vi "Periodic Tasks.vi"(8 "error in":errorcluster) -> (0 "error out":errorcluster)   [LabVIEW 2018]
doc: "This VI runs in parallel to other tasks. It can contain as many user-defined periodic loops as you need. These can carry out PID or other sorts of timed response."
uses:
  <vilib>/Rock Robotics/WPI/Joystick/WPI_JoystickDevRef.ctl
  <vilib>/Rock Robotics/WPI/Joystick/WPI_JoystickDeviceEnum.ctl
  <vilib>/Rock Robotics/WPI/RobotDrive/WPI_RobotDriveDevRef.ctl
  <vilib>/Rock Robotics/WPI/MotorControl/WPI_MotorControlDeviceRef.ctl
  <vilib>/Rock Robotics/WPI/MotorControl/WPI_MotorControlType.ctl
  <vilib>/Rock Robotics/SystemInterfaces/DIO/FPGA_DIOPWMChannel.ctl
  <vilib>/Rock Robotics/WPI/PWM/WPI_PWMDeadband.ctl
  <vilib>/Rock Robotics/SystemInterfaces/DIO/FPGA_DIOChannel.ctl
  <vilib>/Rock Robotics/WPI/Solenoid/WPI_SolenoidDevRef.ctl
  <vilib>/Rock Robotics/WPI/Solenoid/WPI_SolenoidChannel.ctl
  <vilib>/Rock Robotics/WPI/DigitalInput/WPI_DigitalInputDevRef.ctl
  Vision States.ctl
  <vilib>/Rock Robotics/WPI/DriverStation/WPI_DriverStationRobotMode2.ctl
  Hatch Retainer States.ctl
  HAB Bk Spd Motor States.ctl
  Hatch Kicking States.ctl
  <vilib>/Rock Robotics/WPI/ThirdParty/Phoenix-LabVIEW/Motor Controller/Controls/CTRE_Phoenix_MotorControl_MotionProfileTrajectoryPoint.ctl
  <vilib>/Rock Robotics/WPI/Utilities/WPI_GetSetVariantRefNum.vi
  <vilib>/Rock Robotics/WPI/ThirdParty/Phoenix-LabVIEW/Motor Controller/Get/CTRE_Phoenix_MotorController_GetQuadratureData.vi
  Robot Global Data.vi
  <vilib>/Rock Robotics/Network Tables/NT Write Number.vi
  <vilib>/Rock Robotics/WPI/ThirdParty/Phoenix-LabVIEW/Motor Controller/Closed Loop/Motion Profile/CTRE_Phoenix_MotorControl_BufferedTrajectoryPointStream_WriteAll.vi
  <vilib>/Rock Robotics/Network Tables/NT Read Number.vi
  <vilib>/Rock Robotics/WPI/Solenoid/WPI_SolenoidValue.ctl
  <vilib>/Rock Robotics/WPI/Solenoid/WPI_SolenoidSetEnum.vi
  <vilib>/addons/control/pid/NI_PID_pid.lvlib
  <vilib>/Rock Robotics/WPI/ThirdParty/Phoenix-LabVIEW/Motor Controller/Controls/CTRE_Phoenix_MotorControl_ControlMode.ctl
  <vilib>/addons/control/pid/pid.llb/PID (DBL).vi
  <vilib>/Rock Robotics/Network Tables/NT Write Boolean.vi
panel:
  in  "HAB3DriveModuleMotorDevRef 2":T1={"DeviceStatus"={"status"=FALSE, "code"=0, "source"=""}, "Type"=enum."PWM", "PWM"={"PWM Channel"=enum."Invalid", "DeadBand"={"Name"="", "maxPositivePwm"=0, "minPositivePwm"=0, "centerPwm"=0, "maxNegativePwm"=0, "minNegativePwm"=0, "angularRange"=0}}, "CAN"={"Device Number"=0, "SetOutput VI Ref"=variant(refnum<vi> refnum), "GetOutput VI Ref"=variant(refnum<vi> refnum), "Enable VI Ref"=variant(refnum<vi> refnum), "Disable VI Ref"=variant(refnum<vi> refnum), "Data"=variant}, "Invert"=FALSE, "DIO PWM"={"PWM \"Enable\" Channel"=enum."Invalid", "DIOChannel"=enum."Invalid", "PWM Rate"=0.0}}
  in  "BkSpdAdjusterMotorDevRef":T1={"DeviceStatus"={"status"=FALSE, "code"=0, "source"=""}, "Type"=enum."PWM", "PWM"={"PWM Channel"=enum."Invalid", "DeadBand"={"Name"="", "maxPositivePwm"=0, "minPositivePwm"=0, "centerPwm"=0, "maxNegativePwm"=0, "minNegativePwm"=0, "angularRange"=0}}, "CAN"={"Device Number"=0, "SetOutput VI Ref"=variant(refnum<vi> refnum), "GetOutput VI Ref"=variant(refnum<vi> refnum), "Enable VI Ref"=variant(refnum<vi> refnum), "Disable VI Ref"=variant(refnum<vi> refnum), "Data"=variant}, "Invert"=FALSE, "DIO PWM"={"PWM \"Enable\" Channel"=enum."Invalid", "DIOChannel"=enum."Invalid", "PWM Rate"=0.0}}
  in  "HABAssisterSolenoidDevRef":T6={"DevStatus"={"status"=FALSE, "code"=0, "source"=""}, "Pneumatics Control Module"=0, "Forward Solenoid Channel"=enum."Invalid", "Reverse Solenoid Channel"=enum."Invalid"}
  out "Right Traj. Pts Array":dbl[][](array[numeric])
  out "Left Traj. Pts Array":dbl[][](array[numeric])
  in  "Back HAB 3 Limit Switch":T8={"DevStatus"={"status"=FALSE, "code"=0, "source"=""}, "DIO Channel"=enum."Invalid"}
  in  "Front HAB 3 Limit Switch":T8={"DevStatus"={"status"=FALSE, "code"=0, "source"=""}, "DIO Channel"=enum."Invalid"}
  in  "BottomRetainerSwitchDevRef":T8={"DevStatus"={"status"=FALSE, "code"=0, "source"=""}, "DIO Channel"=enum."Invalid"}
  in  "TopRetainerSwitchDevRef":T8={"DevStatus"={"status"=FALSE, "code"=0, "source"=""}, "DIO Channel"=enum."Invalid"}
  in  "HatchRetainerMotorDevRef":T1={"DeviceStatus"={"status"=FALSE, "code"=0, "source"=""}, "Type"=enum."PWM", "PWM"={"PWM Channel"=enum."Invalid", "DeadBand"={"Name"="", "maxPositivePwm"=0, "minPositivePwm"=0, "centerPwm"=0, "maxNegativePwm"=0, "minNegativePwm"=0, "angularRange"=0}}, "CAN"={"Device Number"=0, "SetOutput VI Ref"=variant(refnum<vi> refnum), "GetOutput VI Ref"=variant(refnum<vi> refnum), "Enable VI Ref"=variant(refnum<vi> refnum), "Disable VI Ref"=variant(refnum<vi> refnum), "Data"=variant}, "Invert"=FALSE, "DIO PWM"={"PWM \"Enable\" Channel"=enum."Invalid", "DIOChannel"=enum."Invalid", "PWM Rate"=0.0}}
  in  "HAB3BackSolenoidDevRef":T6={"DevStatus"={"status"=FALSE, "code"=0, "source"=""}, "Pneumatics Control Module"=0, "Forward Solenoid Channel"=enum."Invalid", "Reverse Solenoid Channel"=enum."Invalid"}
  in  "HAB3FrontSolenoidDevRef":T6={"DevStatus"={"status"=FALSE, "code"=0, "source"=""}, "Pneumatics Control Module"=0, "Forward Solenoid Channel"=enum."Invalid", "Reverse Solenoid Channel"=enum."Invalid"}
  in  "AuxJoystickDevRef":T9={"Device"=enum."USB 1"}
  in  "DriveJoystickDevRef":T9={"Device"=enum."USB 1"}
  in  "HAB3DriveModuleMotorDevRef":T1={"DeviceStatus"={"status"=FALSE, "code"=0, "source"=""}, "Type"=enum."PWM", "PWM"={"PWM Channel"=enum."Invalid", "DeadBand"={"Name"="", "maxPositivePwm"=0, "minPositivePwm"=0, "centerPwm"=0, "maxNegativePwm"=0, "minNegativePwm"=0, "angularRange"=0}}, "CAN"={"Device Number"=0, "SetOutput VI Ref"=variant(refnum<vi> refnum), "GetOutput VI Ref"=variant(refnum<vi> refnum), "Enable VI Ref"=variant(refnum<vi> refnum), "Disable VI Ref"=variant(refnum<vi> refnum), "Data"=variant}, "Invert"=FALSE, "DIO PWM"={"PWM \"Enable\" Channel"=enum."Invalid", "DIOChannel"=enum."Invalid", "PWM Rate"=0.0}}
  in  "LifterSolenoidDevRef":T6={"DevStatus"={"status"=FALSE, "code"=0, "source"=""}, "Pneumatics Control Module"=0, "Forward Solenoid Channel"=enum."Invalid", "Reverse Solenoid Channel"=enum."Invalid"}
  in  "DriveJoystickDevRef":T9={"Device"=enum."USB 1"}
  in  "HatchCollectorMotorDevRef":T1={"DeviceStatus"={"status"=FALSE, "code"=0, "source"=""}, "Type"=enum."PWM", "PWM"={"PWM Channel"=enum."Invalid", "DeadBand"={"Name"="", "maxPositivePwm"=0, "minPositivePwm"=0, "centerPwm"=0, "maxNegativePwm"=0, "minNegativePwm"=0, "angularRange"=0}}, "CAN"={"Device Number"=0, "SetOutput VI Ref"=variant(refnum<vi> refnum), "GetOutput VI Ref"=variant(refnum<vi> refnum), "Enable VI Ref"=variant(refnum<vi> refnum), "Disable VI Ref"=variant(refnum<vi> refnum), "Data"=variant}, "Invert"=FALSE, "DIO PWM"={"PWM \"Enable\" Channel"=enum."Invalid", "DIOChannel"=enum."Invalid", "PWM Rate"=0.0}}
  in  "AuxJoystickDevRef":T9
  in  "RetainerSolenoidDevRef":T6={"DevStatus"={"status"=FALSE, "code"=0, "source"=""}, "Pneumatics Control Module"=0, "Forward Solenoid Channel"=enum."Invalid", "Reverse Solenoid Channel"=enum."Invalid"}
  in  "KickerSolenoidDevRef":T6={"DevStatus"={"status"=FALSE, "code"=0, "source"=""}, "Pneumatics Control Module"=0, "Forward Solenoid Channel"=enum."Invalid", "Reverse Solenoid Channel"=enum."Invalid"}
  in  "Drive Motors":T11={"DevStatus"={"status"=FALSE, "code"=0, "source"=""}, "Motors[]"=[], "Square Inputs"=FALSE, "Max Output"=1.0}
  in  "AuxJoystickDevRef":T9={"Device"=enum."USB 1"}
  in  "DriveJoystickDevRef":T9
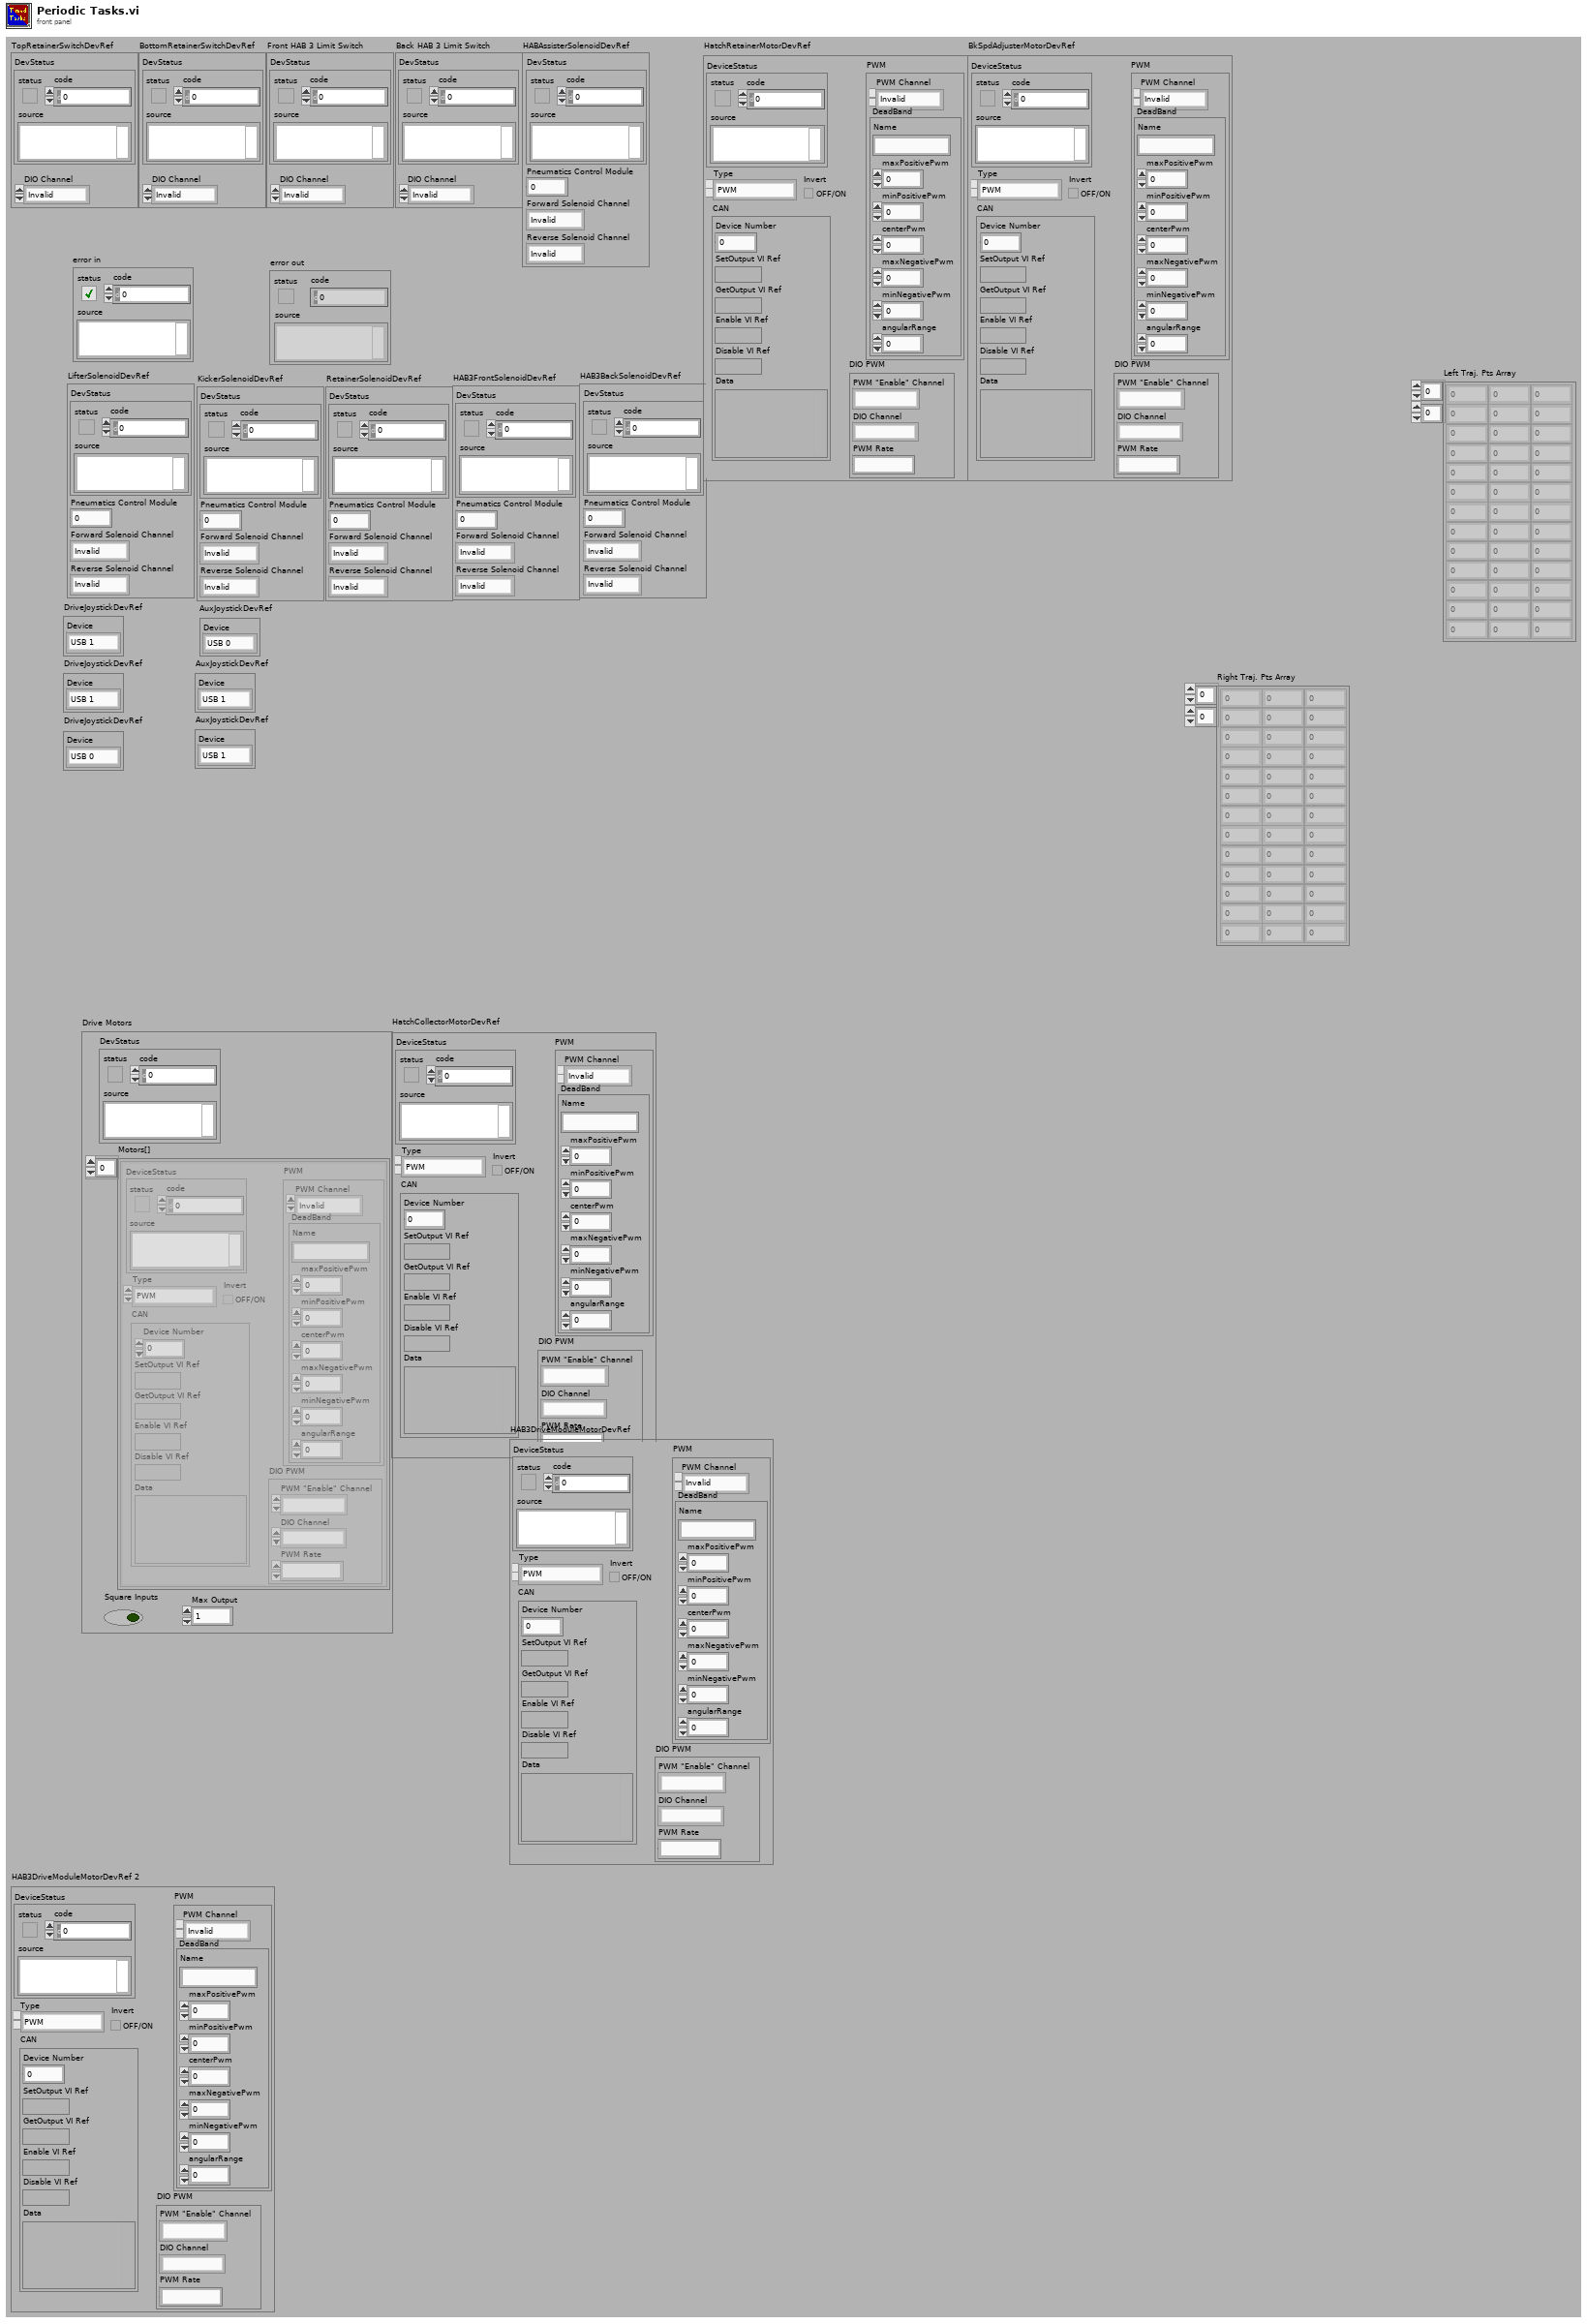
[diagram p1: front panel]
types:
  T1 = typedef "WPI_MotorControlDeviceRef.ctl" = cluster{"DeviceStatus":errorcluster, "Type":T2, "PWM":cluster{"PWM Channel":T3, "DeadBand":T4}, "CAN":cluster{"Device Number":u8, "SetOutput VI Ref":variant, "GetOutput VI Ref":variant, "Enable VI Ref":variant, "Disable VI Ref":variant, "Data":variant}, "Invert":bool, "DIO PWM":cluster{"PWM \"Enable\" Channel":T3, "DIOChannel":T5, "PWM Rate":dbl}}
  T2 = typedef "WPI_MotorControlType.ctl" = enum16{"PWM", "CAN", "DIO PWM"}
  T3 = typedef "FPGA_DIOPWMChannel.ctl" = enum8{"PWM 0", "PWM 1", "PWM 2", "PWM 3", "PWM 4", "PWM 5", "PWM 6", "PWM 7", "PWM 8", "PWM 9", "PWM MXP 0", "PWM MXP 1", "PWM MXP 2", "PWM MXP 3", "PWM MXP 4", "PWM MXP 5", "PWM MXP 6", "PWM MXP 7", "PWM MXP 8", "PWM MXP 9", "Invalid"}
  T4 = typedef "WPI_PWMDeadband.ctl" = cluster{"Name":string, "maxPositivePwm":i32, "minPositivePwm":i32, "centerPwm":i32, "maxNegativePwm":i32, "minNegativePwm":i32, "angularRange":u16}
  T5 = typedef "FPGA_DIOChannel.ctl" = enum8{"DIO 0", "DIO 1", "DIO 2", "DIO 3", "DIO 4", "DIO 5", "DIO 6", "DIO 7", "DIO 8", "DIO 9", "DIO MXP 0", "DIO MXP 1", "DIO MXP 2", "DIO MXP 3", "DIO MXP 4", "DIO MXP 5", "DIO MXP 6", "DIO MXP 7", "DIO MXP 8", "DIO MXP 9", "DIO MXP 10", "DIO MXP 11", "DIO MXP 12", "DIO MXP 13", "DIO MXP 14", "DIO MXP 15", "SPI Port CS1", "SPI Port CS2", "SPI Port CS3", "SPI Port MISO", "SPI Port MOSI", "Invalid"}
  T6 = typedef "WPI_SolenoidDevRef.ctl" = cluster{"DevStatus":errorcluster, "Pneumatics Control Module":u8, "Forward Solenoid Channel":T7, "Reverse Solenoid Channel":T7}
  T7 = typedef "WPI_SolenoidChannel.ctl" = enum8{"Solenoid 0", "Solenoid 1", "Solenoid 2", "Solenoid 3", "Solenoid 4", "Solenoid 5", "Solenoid 6", "Solenoid 7", "Invalid"}
  T8 = typedef "WPI_DigitalInputDevRef.ctl" = cluster{"DevStatus":errorcluster, "DIO Channel":T5}
  T9 = typedef "WPI_JoystickDevRef.ctl" = cluster{"Device":T10}
  T10 = typedef "WPI_JoystickDeviceEnum.ctl" = enum16{"USB 0", "USB 1", "USB 2", "USB 3", "USB 4", "USB 5"}
  T11 = typedef "WPI_RobotDriveDevRef.ctl" = cluster{"DevStatus":errorcluster, "Motors[]":T1[], "Square Inputs":bool, "Max Output":dbl}
  T12 = typedef "Hatch Kicking States.ctl" = enum16{"Ready", "Stop Retaining Hatch", "Kick Hatch"}
  T13 = typedef "HAB Bk Spd Motor States.ctl" = enum16{"Fully Up", "Going Down", "Fully Down", "Going Up"}
  T14 = typedef "Hatch Retainer States.ctl" = enum16{"Fully Down (not retained)", "Going Up", "Fully Up (retained)", "Going Down"}
  T15 = cluster{"X Button":i32, "A Button":i32, "B Button":i32, "Y Button":i32, "LB Button":i32, "RB Button":i32, "LT Button":i32, "RT Button":i32, "BACK Button":i32, "START Button":i32, "LJ Click Button":i32, "RJ Click Button":i32}
  T16 = cluster{"Left X":i32, "Left Y":i32, "Right X":i32, "Right Y":i32}
  T17 = typedef "WPI_DriverStationRobotMode2.ctl" = enum16{"Autonomous Disabled", "Autonomous Enabled", "Teleop Disabled", "Teleop Enabled", "Disconnected", "Finish", "Test Disabled", "Test Enabled", "Emergency Stopped"}
  T18 = cluster{"offsetAngle H":dbl, "offsetAngle V":dbl, "area":dbl, "skew":dbl, "shortest side (pxls)":dbl, "longest side (pxls)":dbl}
  T19 = typedef "Vision States.ctl" = enum16{"Ready", "Forward Until Target at Edge", "Vision Track"}
  T20 = cluster{"A Button":i32, "B Button":i32, "X Button":i32, "Y Button":i32, "LB Button":i32, "RB Button":i32, "BACK Button":i32, "START Button":i32, "LJ Click Button":i32, "RJ Click Button":i32}
  T21 = cluster{"Left X":i32, "Left Y":i32, "Right X":i32, "Right Y":i32, "RT Button":i32, "LT Button":i32}
  T22 = typedef "WPI_GyroDevRef.ctl" = cluster{"DevStatus":errorcluster, "Analog Channel":T23, "Gain (VoltsPerDegree/Second)":dbl, "Gyro Type":enum16{"Analog", "XRS450"}, "Handle":i32, "SPI Bus":T24, "Device Found":bool, "Sample Rate":dbl, "Calibrate On Open":bool, "Offset":dbl}
  T23 = typedef "FPGA_AIChannel.ctl" = enum8{"AI 0", "AI 1", "AI 2", "AI 3", "AI MXP 0", "AI MXP 1", "AI MXP 2", "AI MXP 3", "Invalid"}
  T24 = typedef "spi_bus.ctl" = enum16{"SPI On-Board, CS0", "SPI On-Board, CS1", "SPI On-Board, CS2", "SPI On-Board, CS3", "SPI MXP", "Invalid"}
  T25 = cluster{"HAB3DriveModuleMotorDevRef 2":T1, "DriveJoystickDevRef":T9, "AuxJoystickDevRef":T9, "Drive Axes":dbl[], "Drive Buttons":bool[], "Drive POVs":i16[], "Aux Axes":dbl[], "Aux Buttons":bool[], "Aux POVs":i16[], "Robot Mode":T17, "Drive Motors":T11, "Drive Axes Indexes":cluster{"Left X":i32, "Left Y":i32, "Right X":i32, "Right Y":i32, "RT Button":i32, "LT Button":i32}, "Drive Button Indexes":cluster{"A Button":i32, "B Button":i32, "X Button":i32, "Y Button":i32, "LB Button":i32, "RB Button":i32, "BACK Button":i32, "START Button":i32, "LJ Click Button":i32, "RJ Click Button":i32}, "Joystick VS Vision Latch":bool, "Vision States":T19, "limelight":cluster{"offsetAngle H":dbl, "offsetAngle V":dbl, "area":dbl, "skew":dbl, "shortest side (pxls)":dbl, "longest side (pxls)":dbl}, "Vision Track Mode Override":bool, "T = Motion Profile, F = Percent Output":bool, "Arcade Drive?":bool, "Start Motion Profile?":bool}
  T26 = cluster{"TopRetainerSwitchDevRef":T8, "BottomRetainerSwitchDevRef":T8, "HatchRetainerMotorDevRef":T1, "LifterSolenoidDevRef":T6, "DriveJoystickDevRef":T9, "KickerSolenoidDevRef":T6, "RetainerSolenoidDevRef":T6, "AuxJoystickDevRef":T9, "HatchCollectorMotorDevRef":T1, "Drive Axes":dbl[], "Drive Buttons":bool[], "Drive POVs":i16[], "Aux Axes":dbl[], "Aux Buttons":bool[], "Aux POVs":i16[], "Robot Mode":T17, "Aux Joystick Indexes":cluster{"Left X":i32, "Left Y":i32, "Right X":i32, "Right Y":i32}, "Aux Button Indexes":cluster{"X Button":i32, "A Button":i32, "B Button":i32, "Y Button":i32, "LB Button":i32, "RB Button":i32, "LT Button":i32, "RT Button":i32, "BACK Button":i32, "START Button":i32, "LJ Click Button":i32, "RJ Click Button":i32}, "Hatch Retainer Move Up/Down":bool, "Hatch Collector Actual Angle":dbl, "Hatch Collector Wanted Angle":dbl, "Hatch Retainer States":T14, "Hatch Kicking States":T12}
  T27 = cluster{"BkSpdAdjusterMotorDevRef":T1, "HABAssisterSolenoidDevRef":T6, "Back HAB 3 Limit Switch":T8, "Front HAB 3 Limit Switch":T8, "HAB3DriveModuleMotorDevRef":T1, "DriveJoystickDevRef":T9, "AuxJoystickDevRef":T9, "HAB3FrontSolenoidDevRef":T6, "HAB3BackSolenoidDevRef":T6, "Drive Axes":dbl[], "Drive Buttons":bool[], "Drive POVs":i16[], "Aux Axes":dbl[], "Aux Buttons":bool[], "Aux POVs":i16[], "Robot Mode":T17, "Aux Joystick Indexes":cluster{"Left X":i32, "Left Y":i32, "Right X":i32, "Right Y":i32}, "Aux Button Indexes":cluster{"X Button":i32, "A Button":i32, "B Button":i32, "Y Button":i32, "LB Button":i32, "RB Button":i32, "LT Button":i32, "RT Button":i32, "BACK Button":i32, "START Button":i32, "LJ Click Button":i32, "RJ Click Button":i32}, "Front Cylinders Latch":bool, "Back Cylinders Latch":bool, "Yaw":dbl, "Pitch":dbl, "Roll":dbl, "HAB Bk Spd Motor States":T13}
  T28 = typedef "CTRE_Phoenix_MotorControl_MotionProfileTrajectoryPoint.ctl" = cluster{"Position":dbl, "Velocity":dbl, "Arbitrary Feed Forward":dbl, "Auxiliary Position":dbl, "Auxiliary Velocity":dbl, "Auxiliary Arbitrary Feed Forward":dbl, "Profile Slot Select":i32, "Auxiliary Profile Slot Select":i32, "isLastPoint?":bool, "Zero Position?":bool, "durationMs":u32, "Use Aux PID?":bool}
  T29 = typedef "Which Robot Enum.ctl" = enum16{"Competition Bot", "Practice Bot", "Code Bot"}
  T30 = typedef "CTRE_Phoenix_MotorControl_BufferedTrajectoryPointStream_DeviceRef.ctl" = cluster{"Handle":u64, "Library Path":path}
  T31 = typedef "WPI_SolenoidValue.ctl" = enum16{"Off", "On", "Forward", "Reverse"}
  T32 = cluster{"proportional gain (Kc)":dbl, "integral time (Ti, min)":dbl, "derivative time (Td, min)":dbl}
  T33 = typedef "CTRE_Phoenix_MotorControl_ControlMode.ctl" = u16
  T34 = cluster{"Yaw":dbl, "Roll":dbl, "Pitch":dbl, "Heading":dbl, "Fused Heading":dbl}
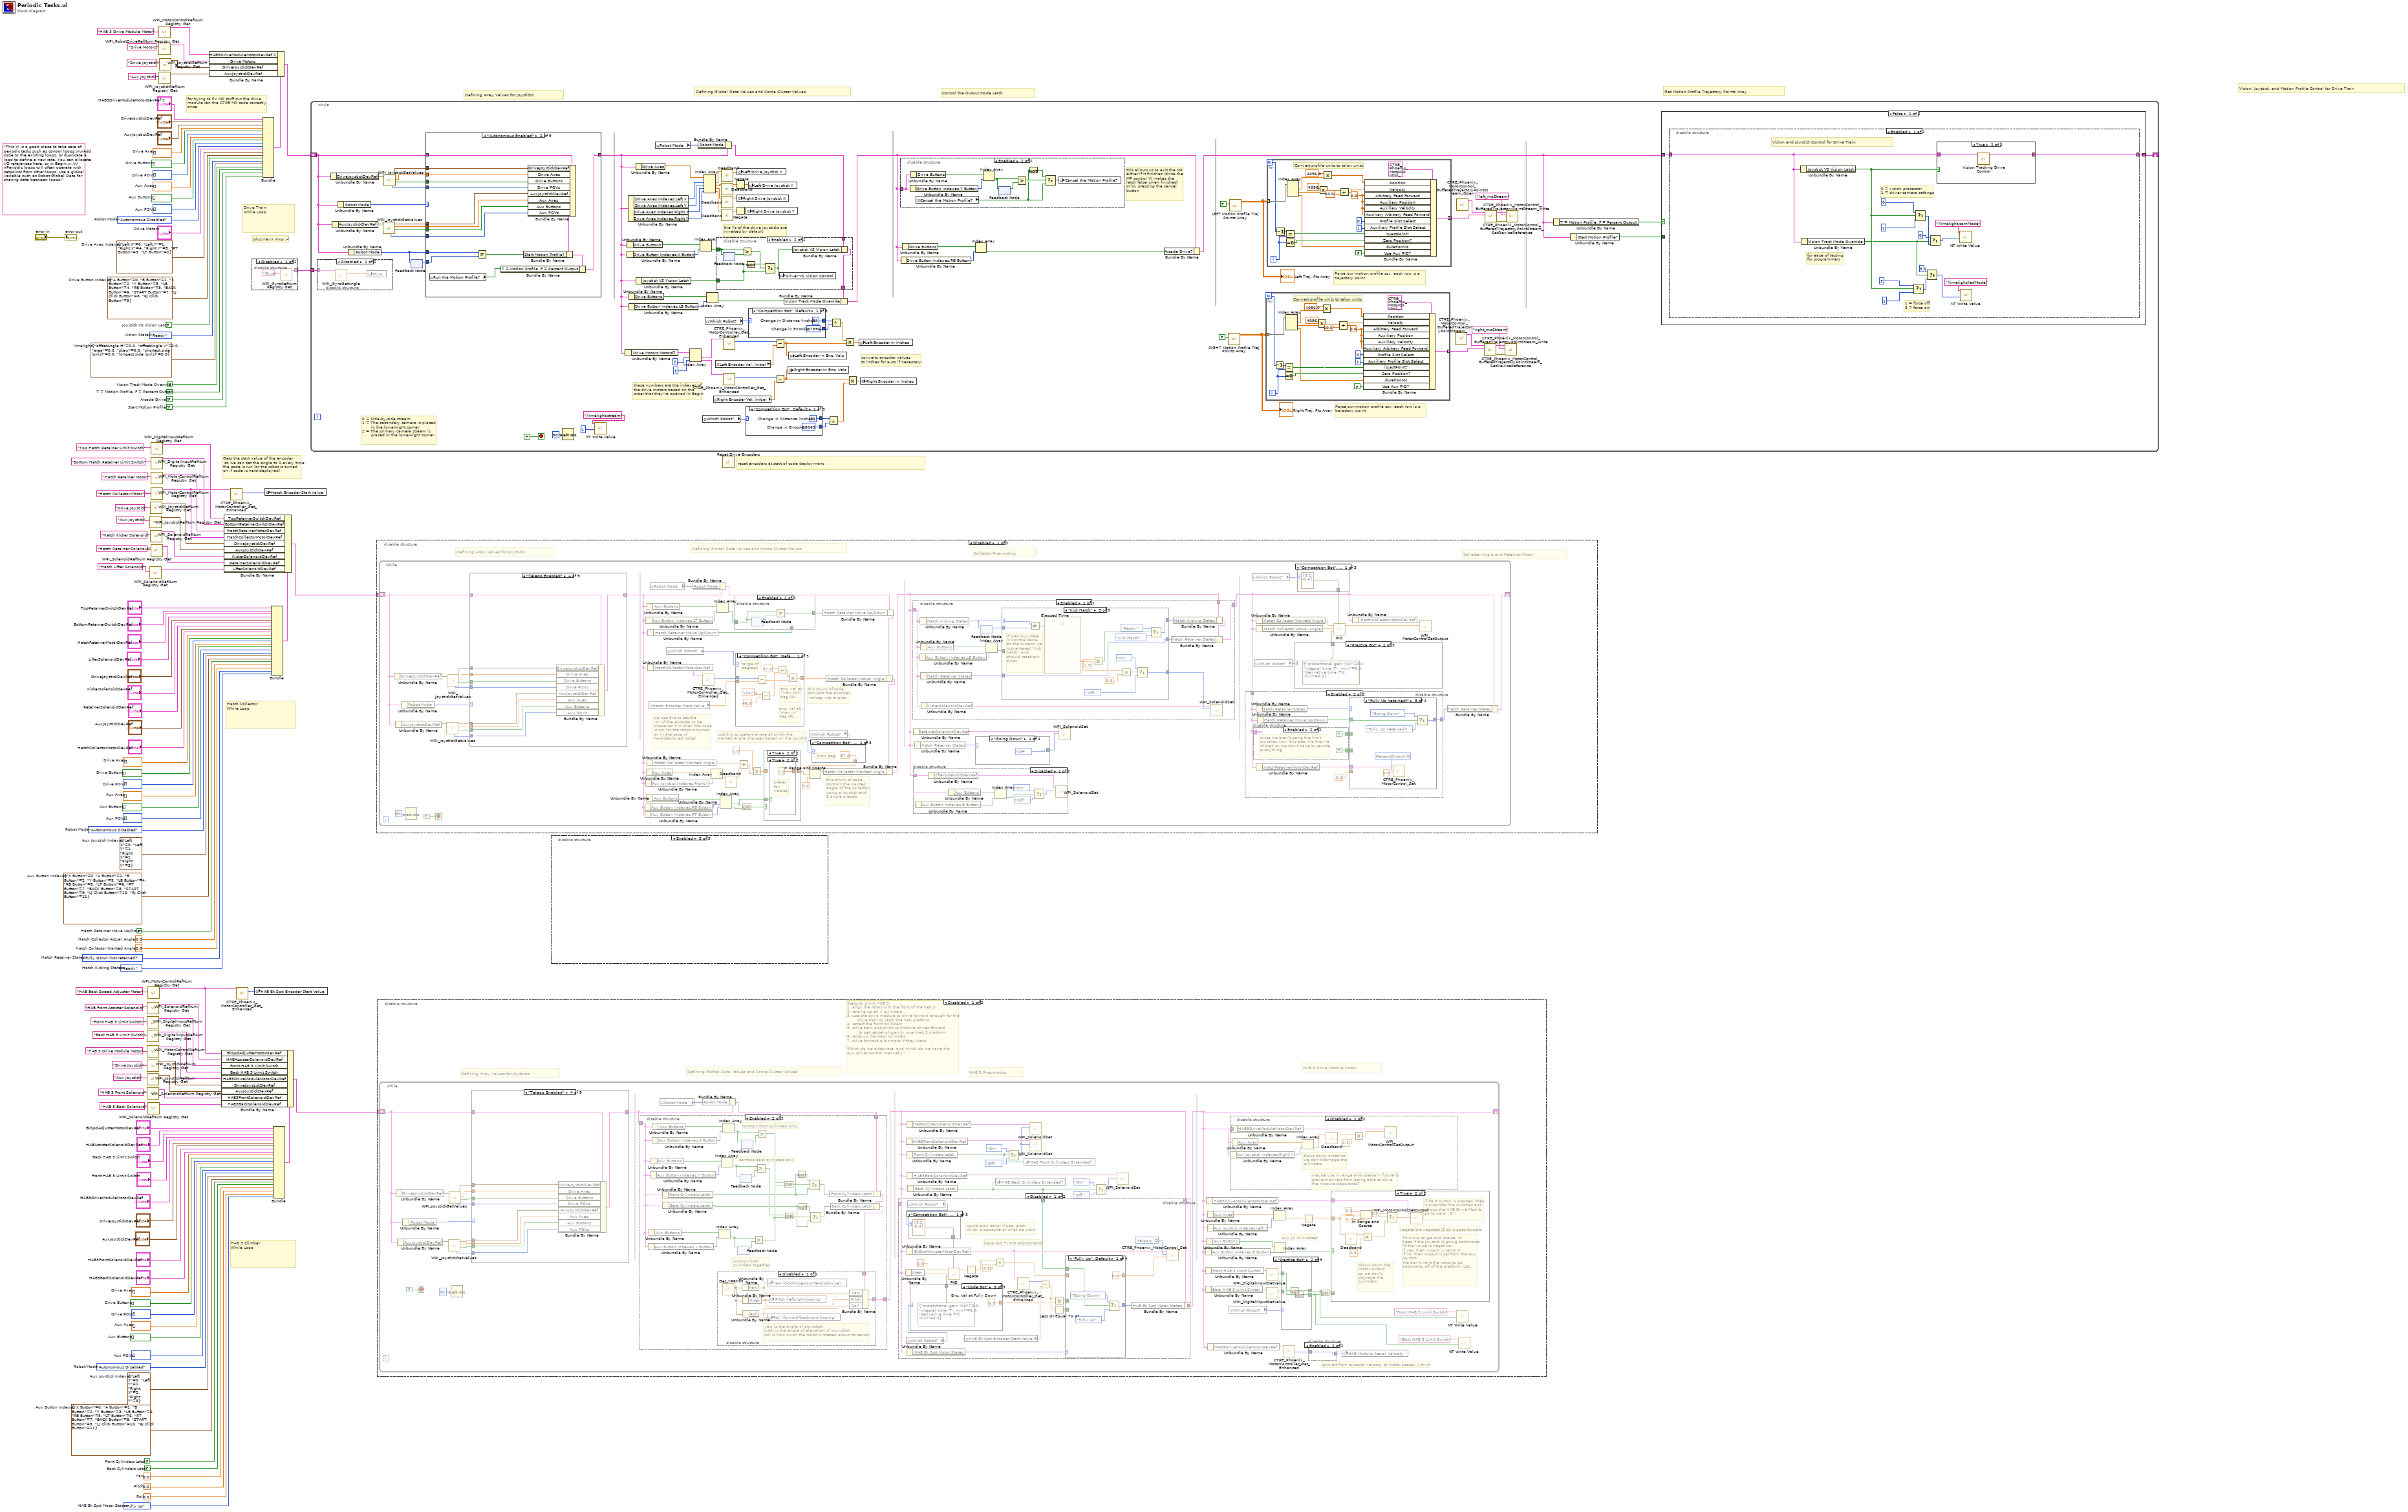
[diagram p0: block diagram]
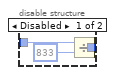
[diagram p2: hidden frame]
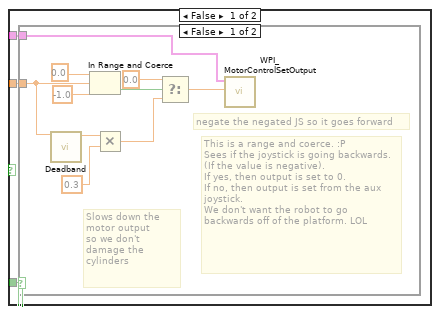
[diagram p3: hidden frame]
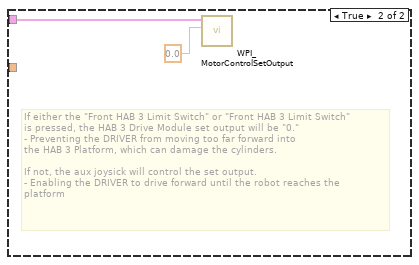
[diagram p4: hidden frame]
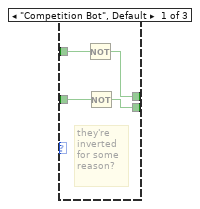
[diagram p5: hidden frame]
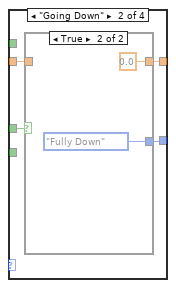
[diagram p7: hidden frame]
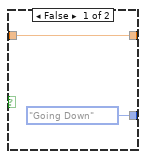
[diagram p8: hidden frame]
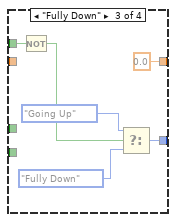
[diagram p9: hidden frame]
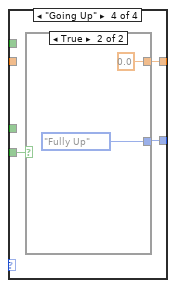
[diagram p10: hidden frame]
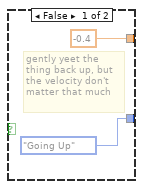
[diagram p11: hidden frame]
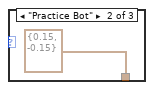
[diagram p12: hidden frame]
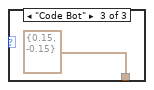
[diagram p13: hidden frame]
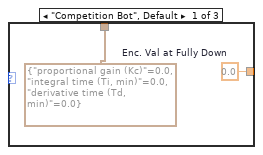
[diagram p14: hidden frame]
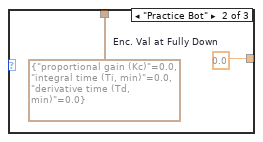
[diagram p15: hidden frame]
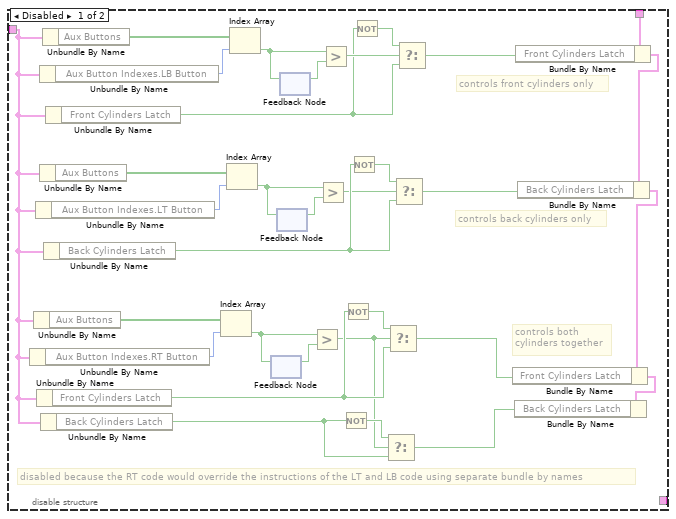
[diagram p17: hidden frame]
diagram:
  w4 = FALSE  # Start Motion Profile?
  w5 = FALSE  # Arcade Drive?
  w6 = Hatch_Kicking_States."Ready"  # Hatch Kicking States
  w7 = HAB_Bk_Spd_Motor_States."Fully Up"  # HAB Bk Spd Motor States
  w12 = 0.0  # Roll
  w13 = 0.0  # Pitch
  w14 = 0.0  # Yaw
  w24 = Hatch_Retainer_States."Fully Down (not retained)"  # Hatch Retainer States
  w34 = FALSE  # T = Motion Profile, F = Percent Output
  w36 = 0.0  # Hatch Collector Wanted Angle
  w37 = FALSE  # Back Cylinders Latch
  w38 = FALSE  # Front Cylinders Latch
  w39 = T15 {"X Button"=0, "A Button"=1, "B Button"=2, "Y Button"=3, "LB Button"=4, "RB Button"=5, "LT Button"=6, "RT Button"=7, "BACK Button"=8, "START Button"=9, "LJ Click Button"=10, "RJ Click Button"=11}  # Aux Button Indexes
  w40 = T16 {"Left X"=0, "Left Y"=1, "Right X"=2, "Right Y"=3}  # Aux Joystick Indexes
  w41 = WPI_DriverStationRobotMode2."Autonomous Disabled"  # Robot Mode
  w42 = i16[] []  # Aux POVs
  w43 = bool[] []  # Aux Buttons
  w44 = dbl[] []  # Aux Axes
  w45 = i16[] []  # Drive POVs
  w46 = bool[] []  # Drive Buttons
  w47 = dbl[] []  # Drive Axes
  w70 = 0.0  # Hatch Collector Actual Angle
  w71 = FALSE  # Hatch Retainer Move Up/Down
  w72 = T15 {"X Button"=0, "A Button"=1, "B Button"=2, "Y Button"=3, "LB Button"=4, "RB Button"=5, "LT Button"=6, "RT Button"=7, "BACK Button"=8, "START Button"=9, "LJ Click Button"=10, "RJ Click Button"=11}  # Aux Button Indexes
  w73 = T16 {"Left X"=0, "Left Y"=1, "Right X"=2, "Right Y"=3}  # Aux Joystick Indexes
  w77 = WPI_DriverStationRobotMode2."Autonomous Disabled"  # Robot Mode
  w78 = i16[] []  # Aux POVs
  w79 = bool[] []  # Aux Buttons
  w80 = dbl[] []  # Aux Axes
  w81 = i16[] []  # Drive POVs
  w82 = bool[] []  # Drive Buttons
  w83 = dbl[] []  # Drive Axes
  w97 = FALSE  # Vision Track Mode Override
  w98 = T18 {"offsetAngle H"=0.0, "offsetAngle V"=0.0, "area"=0.0, "skew"=0.0, "shortest side (pxls)"=0.0, "longest side (pxls)"=0.0}  # limelight
  w99 = Vision_States."Ready"  # Vision States
  w100 = FALSE  # Joystick VS Vision Latch
  w101 = T20 {"A Button"=0, "B Button"=1, "X Button"=2, "Y Button"=3, "LB Button"=4, "RB Button"=5, "BACK Button"=6, "START Button"=7, "LJ Click Button"=8, "RJ Click Button"=9}  # Drive Button Indexes
  w103 = T21 {"Left X"=0, "Left Y"=1, "Right X"=4, "Right Y"=5, "RT Button"=3, "LT Button"=2}  # Drive Axes Indexes
  w108 = i16[] []  # Aux POVs
  w109 = bool[] []  # Aux Buttons
  w110 = dbl[] []  # Aux Axes
  w107 = WPI_DriverStationRobotMode2."Autonomous Disabled"  # Robot Mode
  w111 = i16[] []  # Drive POVs
  w112 = bool[] []  # Drive Buttons
  w113 = dbl[] []  # Drive Axes
  (unwired) "This VI is a good place to take care of periodic tasks such as control loops.\n\nAdd code to the existing loops, or duplicate a loop to define a new rate. You can allocate I/O references here, or in Begin.vi.\n\nPeriodic loops will often operate with setpoints from other loops. Use a global variable such as Robot Global Data for sharing data between loops."
  # "for trying to fix MP stuff cuz the drive\nmodule ran the CTRE MP code correctly\nonce"
  # "reset encoders at start of code deployment"
  # "Get Motion Profile Trajectory Points Array"
  # "Control the Output Mode Latch"
  # "plus navX mxp :-)"
  # "Gets the start value of the encoder\n so we can set the angle to 0 every time\nthe code is run (or the robot is turned\non if code is hard-deployed)"
  # "HAB 3 Climber\nWhile Loop"
  # "Hatch Collector\nWhile Loop"
  # "Drive Train\nWhile Loop"
  # "Vision, Joystick, and Motion Profile Control for Drive Train"
  # "Defining Array Values for Joysticks"
  # "Defining Global Data Values and Some Cluster Values"
  n1 = call <vilib>:"WPI_DigitalInputRefNum Registry Get.vi"("refnum name"="Front HAB 3 Limit Switch") -> ("DigitalInputDevRef"=w19:T8)  [unwired: 9 in, 1 out]
  n2 = call <vilib>:"WPI_JoystickRefNum Registry Get.vi"("refnum name"="Aux Joystick") -> ("JoystickDevRef"=w51:T9)  [unwired: 9 in, 1 out]
  n3 = call <vilib>:"WPI_SolenoidRefNum Registry Get.vi"("refnum name"="HAB Front Assister Solenoid") -> ("SolenoidDevRef"=w15:T6)  [unwired: 9 in, 1 out]
  n4 = call <vilib>:"WPI_DigitalInputRefNum Registry Get.vi"("refnum name"="Back HAB 3 Limit Switch") -> ("DigitalInputDevRef"=w18:T8)  [unwired: 9 in, 1 out]
  n5 = call <vilib>:"WPI_MotorControlRefNum Registry Get.vi"("refnum name"="HAB 3 Drive Module Motor") -> ("MotorControlDevRef"=w49:T1)  [unwired: 9 in, 1 out]
  n6 = call <vilib>:"WPI_JoystickRefNum Registry Get.vi"("refnum name"="Drive Joystick") -> ("JoystickDevRef"=w50:T9)  [unwired: 9 in, 1 out]
  n7 = call <vilib>:"WPI_SolenoidRefNum Registry Get.vi"("refnum name"="HAB 3 Front Solenoid") -> ("SolenoidDevRef"=w52:T6)  [unwired: 9 in, 1 out]
  n8 = call <vilib>:"WPI_MotorControlRefNum Registry Get.vi"("refnum name"="HAB Back Speed Adjuster Motor") -> ("MotorControlDevRef"=w8:T1)  [unwired: 9 in, 1 out]
  n9 = call <vilib>:"WPI_SolenoidRefNum Registry Get.vi"("refnum name"="HAB 3 Back Solenoid") -> ("SolenoidDevRef"=w53:T6)  [unwired: 9 in, 1 out]
  n10 = call <vilib>:"WPI_SolenoidRefNum Registry Get.vi"("refnum name"="Hatch Lifter Solenoid") -> ("SolenoidDevRef"=w66:T6)  [unwired: 9 in, 1 out]
  n11 = call <vilib>:"WPI_JoystickRefNum Registry Get.vi"("refnum name"="Aux Joystick") -> ("JoystickDevRef"=w88:T9)  [unwired: 9 in, 1 out]
  n12 = call <vilib>:"WPI_JoystickRefNum Registry Get.vi"("refnum name"="Drive Joystick") -> ("JoystickDevRef"=w74:T9)  [unwired: 9 in, 1 out]
  n13 = call <vilib>:"WPI_SolenoidRefNum Registry Get.vi"("refnum name"="Hatch Kicker Solenoid") -> ("SolenoidDevRef"=w91:T6)  [unwired: 9 in, 1 out]
  n14 = call <vilib>:"WPI_SolenoidRefNum Registry Get.vi"("refnum name"="Hatch Retainer Solenoid") -> ("SolenoidDevRef"=w90:T6)  [unwired: 9 in, 1 out]
  n15 = call <vilib>:"WPI_DigitalInputRefNum Registry Get.vi"("refnum name"="Top Hatch Retainer Limit Switch") -> ("DigitalInputDevRef"=w25:T8)  [unwired: 9 in, 1 out]
  n16 = call <vilib>:"WPI_DigitalInputRefNum Registry Get.vi"("refnum name"="Bottom Hatch Retainer Limit Switch") -> ("DigitalInputDevRef"=w26:T8)  [unwired: 9 in, 1 out]
  n17 = call <vilib>:"WPI_MotorControlRefNum Registry Get.vi"("refnum name"="Hatch Retainer Motor") -> ("MotorControlDevRef"=w31:T1)  [unwired: 9 in, 1 out]
  n18 = call <vilib>:"WPI_MotorControlRefNum Registry Get.vi"("refnum name"="Hatch Collector Motor") -> ("MotorControlDevRef"=w69:T1)  [unwired: 9 in, 1 out]
  n19 = call <vilib>:"WPI_MotorControlRefNum Registry Get.vi"("refnum name"="HAB 3 Drive Module Motor") -> ("MotorControlDevRef"=w1:T1)  [unwired: 9 in, 1 out]
  n20 = call <vilib>:"WPI_RobotDriveRefNum Registry Get.vi"("refnum name"="Drive Motors") -> ("RobotDriveDevRef"=w105:T11)  [unwired: 9 in, 1 out]
  n21 = call <vilib>:"WPI_JoystickRefNum Registry Get.vi"("refnum name"="Aux Joystick") -> ("JoystickDevRef"=w115:T9)  [unwired: 9 in, 1 out]
  n22 = call <vilib>:"WPI_JoystickRefNum Registry Get.vi"("refnum name"="Drive Joystick") -> ("JoystickDevRef"=w116:T9)  [unwired: 9 in, 1 out]
  n23 = call-poly <vilib>:"CTRE_Phoenix_MotorController_Get_Enhanced.vi"("PhoenixMotorControlDevRef"=w69) -> ("Quadrature Position"=w68:i32)  [unwired: 11 in, 3 out]
  n24 = call-poly <vilib>:"CTRE_Phoenix_MotorController_Get_Enhanced.vi"("PhoenixMotorControlDevRef"=w8) -> ("Quadrature Position"=w9:i32)  [unwired: 11 in, 3 out]
  n25 = disable-structure shown="Disabled" {
    disable-tunnel: [w122 _] -> w35
    frame Disabled {
      n26 = call <vilib>:"WPI_GyroRefNum Registry Get.vi"("refnum name"="Gyro") -> ("GyroDevRef"=w122:T22)  [unwired: 9 in, 1 out]
    }
    frame Enabled {
    }
  }
  n27 = global write "Robot Global Data.vi" "HAB Bk Spd Encoder Start Value"(w9) -> ()
  n28 = Bundle("HAB3DriveModuleMotorDevRef 2"="HAB3DriveModuleMotorDevRef 2", "DriveJoystickDevRef"="DriveJoystickDevRef", "AuxJoystickDevRef"="AuxJoystickDevRef", "Drive Axes"=w113, "Drive Buttons"=w112, "Drive POVs"=w111, "Aux Axes"=w110, "Aux Buttons"=w109, "Aux POVs"=w108, "Robot Mode"=w107, "Drive Motors"="Drive Motors", "Drive Axes Indexes"=w103, "Drive Button Indexes"=w101, "Joystick VS Vision Latch"=w100, "Vision States"=w99, "limelight"=w98, "Vision Track Mode Override"=w97, "T = Motion Profile, F = Percent Output"=w34, "Arcade Drive?"=w5, "Start Motion Profile?"=w4) -> (w117:T25)  [unwired: 1 in]
  n29 = Bundle By Name(cluster=w117, "HAB3DriveModuleMotorDevRef 2"=w1, "Drive Motors"=w105, "DriveJoystickDevRef"=w116, "AuxJoystickDevRef"=w115) -> (w114:T25)
  n30 = global write "Robot Global Data.vi" "Hatch Encoder Start Value"(w68) -> ()
  n31 = Bundle("TopRetainerSwitchDevRef"="TopRetainerSwitchDevRef", "BottomRetainerSwitchDevRef"="BottomRetainerSwitchDevRef", "HatchRetainerMotorDevRef"="HatchRetainerMotorDevRef", "LifterSolenoidDevRef"="LifterSolenoidDevRef", "DriveJoystickDevRef"="DriveJoystickDevRef", "KickerSolenoidDevRef"="KickerSolenoidDevRef", "RetainerSolenoidDevRef"="RetainerSolenoidDevRef", "AuxJoystickDevRef"="AuxJoystickDevRef", "HatchCollectorMotorDevRef"="HatchCollectorMotorDevRef", "Drive Axes"=w83, "Drive Buttons"=w82, "Drive POVs"=w81, "Aux Axes"=w80, "Aux Buttons"=w79, "Aux POVs"=w78, "Robot Mode"=w77, "Aux Joystick Indexes"=w73, "Aux Button Indexes"=w72, "Hatch Retainer Move Up/Down"=w71, "Hatch Collector Actual Angle"=w70, "Hatch Collector Wanted Angle"=w36, "Hatch Retainer States"=w24, "Hatch Kicking States"=w6) -> (w94:T26)  [unwired: 1 in]
  n32 = Bundle By Name(cluster=w94, "TopRetainerSwitchDevRef"=w25, "BottomRetainerSwitchDevRef"=w26, "HatchRetainerMotorDevRef"=w31, "HatchCollectorMotorDevRef"=w69, "DriveJoystickDevRef"=w74, "AuxJoystickDevRef"=w88, "KickerSolenoidDevRef"=w91, "RetainerSolenoidDevRef"=w90, "LifterSolenoidDevRef"=w66) -> (w84:T26)
  n33 = Bundle("BkSpdAdjusterMotorDevRef"="BkSpdAdjusterMotorDevRef", "HABAssisterSolenoidDevRef"="HABAssisterSolenoidDevRef", "Back HAB 3 Limit Switch"="Back HAB 3 Limit Switch", "Front HAB 3 Limit Switch"="Front HAB 3 Limit Switch", "HAB3DriveModuleMotorDevRef"="HAB3DriveModuleMotorDevRef", "DriveJoystickDevRef"="DriveJoystickDevRef", "AuxJoystickDevRef"="AuxJoystickDevRef", "HAB3FrontSolenoidDevRef"="HAB3FrontSolenoidDevRef", "HAB3BackSolenoidDevRef"="HAB3BackSolenoidDevRef", "Drive Axes"=w47, "Drive Buttons"=w46, "Drive POVs"=w45, "Aux Axes"=w44, "Aux Buttons"=w43, "Aux POVs"=w42, "Robot Mode"=w41, "Aux Joystick Indexes"=w40, "Aux Button Indexes"=w39, "Front Cylinders Latch"=w38, "Back Cylinders Latch"=w37, "Yaw"=w14, "Pitch"=w13, "Roll"=w12, "HAB Bk Spd Motor States"=w7) -> (w54:T27)  [unwired: 1 in]
  n34 = Bundle By Name(cluster=w54, "BkSpdAdjusterMotorDevRef"=w8, "HABAssisterSolenoidDevRef"=w15, "Front HAB 3 Limit Switch"=w19, "Back HAB 3 Limit Switch"=w18, "HAB3DriveModuleMotorDevRef"=w49, "DriveJoystickDevRef"=w50, "AuxJoystickDevRef"=w51, "HAB3FrontSolenoidDevRef"=w52, "HAB3BackSolenoidDevRef"=w53) -> (w48:T27)
  n35 = while {
    shift-right: [w210] -> _
    shift-left: w114 -> [w129]
    tunnel: w35 -> [w172]
    stop <- FALSE stop-if-true
    # "0 = Side-by-side stream\n1 = The secondary camera is placed\n       in the lower-right corner\n2 = The primary camera stream is\n       placed in the lower-right corner"
    # "converts encoder values\nto inches for auto if necessary"
    # "Parse our motion profile csv, each row is a trajectory point"
    # "Parse our motion profile csv, each row is a trajectory point"
    # "this allows us to exit the MP \neither if it finishes (since the\nMP control VI makes the\nlatch false when finished) \nor by pressing the cancel \nbutton"
    # "these numbers are the indexes of\nthe drive motors based on the\norder that they're opened in Begin"
    # "the Ys of the drive joysticks are \ninverted by default"
    n36 = disable-structure shown="Disabled" {
      disable-tunnel: w172 -> [w378 _]
      frame Disabled {
        n37 = call <vilib>:"WPI_GyroGetAngle.vi"("GyroDevRef"=w378) -> ("Angle"=w379:dbl)  [unwired: 6 in, 4 out]
        n38 = global write "Robot Global Data.vi" "Gyro"(w379) -> ()
      }
      frame Enabled {
      }
    }
    n39 = Unbundle By Name(w129) -> ("DriveJoystickDevRef"=w208:T9)
    n40 = Unbundle By Name(w129) -> ("AuxJoystickDevRef"=w207:T9)
    n41 = Unbundle By Name(w129) -> ("Robot Mode"=w206:T17)
    n42 = Unbundle By Name(w129) -> ("Robot Mode"=w128:T17)
    n43 = call <vilib>:"WPI_JoystickGetValues.vi"("JoystickDevRef"=w207) -> ("Buttons"=w199:bool[], "Axes"=w200:dbl[], "JoystickDevRef"=w201:T9, "POVs"=w198:i16[])  [unwired: 6 in, 1 out]
    n44 = call <vilib>:"WPI_JoystickGetValues.vi"("JoystickDevRef"=w208) -> ("Buttons"=w203:bool[], "Axes"=w205:dbl[], "JoystickDevRef"=w204:T9, "POVs"=w202:i16[])  [unwired: 6 in, 1 out]
    n45 = feedback #1() -> (w127:T17)  [unwired: 1 in]
    n46 = feedback-in #1(w128) -> ()
    n47 = case shown="\"Autonomous Enabled\"" w206 {
      tunnel: w129 -> [w396 w418 w424 w444 w450 w462 w474 w494 w500]
      tunnel: [w392 w404 w419 w431 w445 w457 w469 w481 w495] -> w171
      tunnel: w205 -> [_ w417 _ w442 _ _ _ w492 _]
      tunnel: w204 -> [_ w416 _ w443 _ _ _ w493 _]
      tunnel: w203 -> [_ w415 _ w441 _ _ _ w491 _]
      tunnel: w202 -> [_ w414 _ w440 _ _ _ w490 _]
      tunnel: w201 -> [_ w413 _ w439 _ _ _ w489 _]
      tunnel: w200 -> [_ w412 _ w438 _ _ _ w488 _]
      tunnel: w199 -> [_ w411 _ w437 _ _ _ w487 _]
      tunnel: w198 -> [_ w410 _ w436 _ _ _ w486 _]
      tunnel: w128 -> [_ w409 _ _ _ _ _ _ _]
      tunnel: w127 -> [_ w408 _ _ _ _ _ _ _]
      frame "Autonomous Disabled", Default {
        n48 = disable-structure shown="Enabled" {
          disable-tunnel: w396 -> [w398 w402]
          disable-tunnel: [w397 w401] -> w394
          frame Disabled {
            n49 = Bundle By Name(cluster=w398, "Joystick VS Vision Latch"=FALSE) -> (w397:T25)
          }
          frame Enabled {
            n50 = Bundle By Name(cluster=w402, "Vision States"=Vision_States."Ready") -> (w401:T25)
          }
        }
        n51 = Bundle By Name(cluster=w394, "Start Motion Profile?"=FALSE ("T = Motion Profile, F = Percent Output")) -> (w393:T25)
        n52 = Bundle By Name(cluster=w393, "T = Motion Profile, F = Percent Output"=FALSE) -> (w392:T25)
      }
      frame "Autonomous Enabled" {
        n53 = global read "Robot Global Data.vi" "Run the Motion Profile?"() -> (w403:bool)
        n54 = Not Equal?(x=w409, y=w408) -> (x != y?=w407:bool)
        n55 = Bundle By Name(cluster=w418, "DriveJoystickDevRef"=w416, "Drive Axes"=w417, "Drive Buttons"=w415, "Drive POVs"=w414, "AuxJoystickDevRef"=w413, "Aux Axes"=w412, "Aux Buttons"=w411, "Aux POVs"=w410) -> (w406:T25)
        n56 = Bundle By Name(cluster=w406, "Start Motion Profile?"=w407) -> (w405:T25)
        n57 = Bundle By Name(cluster=w405, "T = Motion Profile, F = Percent Output"=w403) -> (w404:T25)
      }
      frame "Teleop Disabled" {
        n58 = disable-structure shown="Enabled" {
          disable-tunnel: w424 -> [w426 w430]
          disable-tunnel: [w425 w429] -> w422
          frame Disabled {
            n59 = Bundle By Name(cluster=w426, "Joystick VS Vision Latch"=FALSE) -> (w425:T25)
          }
          frame Enabled {
            n60 = Bundle By Name(cluster=w430, "Vision States"=Vision_States."Ready") -> (w429:T25)
          }
        }
        n61 = Bundle By Name(cluster=w422, "Start Motion Profile?"=FALSE ("T = Motion Profile, F = Percent Output")) -> (w420:T25)
        n62 = Bundle By Name(cluster=w420, "T = Motion Profile, F = Percent Output"=FALSE) -> (w419:T25)
      }
      frame "Teleop Enabled" {
        n63 = Bundle By Name(cluster=w444, "DriveJoystickDevRef"=w443, "Drive Axes"=w442, "Drive Buttons"=w441, "Drive POVs"=w440, "AuxJoystickDevRef"=w439, "Aux Axes"=w438, "Aux Buttons"=w437, "Aux POVs"=w436) -> (w435:T25)
        n64 = Bundle By Name(cluster=w435, "Start Motion Profile?"=FALSE ("T = Motion Profile, F = Percent Output")) -> (w432:T25)
        n65 = Bundle By Name(cluster=w432, "T = Motion Profile, F = Percent Output"=FALSE) -> (w431:T25)
      }
      frame "Disconnected" {
        n66 = disable-structure shown="Enabled" {
          disable-tunnel: w450 -> [w452 w456]
          disable-tunnel: [w451 w455] -> w448
          frame Disabled {
            n67 = Bundle By Name(cluster=w452, "Joystick VS Vision Latch"=FALSE) -> (w451:T25)
          }
          frame Enabled {
            n68 = Bundle By Name(cluster=w456, "Vision States"=Vision_States."Ready") -> (w455:T25)
          }
        }
        n69 = Bundle By Name(cluster=w448, "Start Motion Profile?"=FALSE ("T = Motion Profile, F = Percent Output")) -> (w446:T25)
        n70 = Bundle By Name(cluster=w446, "T = Motion Profile, F = Percent Output"=FALSE) -> (w445:T25)
      }
      frame "Finish" {
        n71 = disable-structure shown="Enabled" {
          disable-tunnel: w462 -> [w464 w468]
          disable-tunnel: [w463 w467] -> w460
          frame Disabled {
            n72 = Bundle By Name(cluster=w464, "Joystick VS Vision Latch"=FALSE) -> (w463:T25)
          }
          frame Enabled {
            n73 = Bundle By Name(cluster=w468, "Vision States"=Vision_States."Ready") -> (w467:T25)
          }
        }
        n74 = Bundle By Name(cluster=w460, "Start Motion Profile?"=FALSE ("T = Motion Profile, F = Percent Output")) -> (w458:T25)
        n75 = Bundle By Name(cluster=w458, "T = Motion Profile, F = Percent Output"=FALSE) -> (w457:T25)
      }
      frame "Test Disabled" {
        n76 = disable-structure shown="Enabled" {
          disable-tunnel: w474 -> [w476 w480]
          disable-tunnel: [w475 w479] -> w472
          frame Disabled {
            n77 = Bundle By Name(cluster=w476, "Joystick VS Vision Latch"=FALSE) -> (w475:T25)
          }
          frame Enabled {
            n78 = Bundle By Name(cluster=w480, "Vision States"=Vision_States."Ready") -> (w479:T25)
          }
        }
        n79 = Bundle By Name(cluster=w472, "Start Motion Profile?"=FALSE ("T = Motion Profile, F = Percent Output")) -> (w470:T25)
        n80 = Bundle By Name(cluster=w470, "T = Motion Profile, F = Percent Output"=FALSE) -> (w469:T25)
      }
      frame "Test Enabled" {
        n81 = Bundle By Name(cluster=w494, "DriveJoystickDevRef"=w493, "Drive Axes"=w492, "Drive Buttons"=w491, "Drive POVs"=w490, "AuxJoystickDevRef"=w489, "Aux Axes"=w488, "Aux Buttons"=w487, "Aux POVs"=w486) -> (w484:T25)
        n82 = Bundle By Name(cluster=w484, "Start Motion Profile?"=FALSE ("T = Motion Profile, F = Percent Output")) -> (w482:T25)
        n83 = Bundle By Name(cluster=w482, "T = Motion Profile, F = Percent Output"=FALSE) -> (w481:T25)
      }
      frame "Emergency Stopped" {
        n84 = disable-structure shown="Enabled" {
          disable-tunnel: w500 -> [w502 w506]
          disable-tunnel: [w501 w505] -> w498
          frame Disabled {
            n85 = Bundle By Name(cluster=w502, "Joystick VS Vision Latch"=FALSE) -> (w501:T25)
          }
          frame Enabled {
            n86 = Bundle By Name(cluster=w506, "Vision States"=Vision_States."Ready") -> (w505:T25)
          }
        }
        n87 = Bundle By Name(cluster=w498, "Start Motion Profile?"=FALSE ("T = Motion Profile, F = Percent Output")) -> (w496:T25)
        n88 = Bundle By Name(cluster=w496, "T = Motion Profile, F = Percent Output"=FALSE) -> (w495:T25)
      }
    }
    n89 = Wait (ms)(milliseconds to wait=u32 50) -> ()  [unwired: 1 out]
    n90 = call-poly <vilib>:"NT Write Value.vi"("Numeric"=1, "Name"="/limelight/stream") -> ()  [unwired: 9 in, 1 out]
    n91 = Unbundle By Name(w171) -> ("Drive Motors.Motors[]"=w170:T1[])
    n92 = Unbundle By Name(w171) -> ("Drive Buttons"=w177:bool[])
    n93 = Unbundle By Name(w171) -> ("Drive Button Indexes.A Button"=w194:i32)
    n94 = Unbundle By Name(w171) -> ("Drive Axes Indexes.Left X"=w179:i32, "Drive Axes Indexes.Left Y"=w180:i32, "Drive Axes Indexes.Right X"=w181:i32, "Drive Axes Indexes.Right Y"=w182:i32)
    n95 = Unbundle By Name(w171) -> ("Drive Buttons"=w176:bool[])
    n96 = Unbundle By Name(w171) -> ("Drive Button Indexes.LB Button"=w175:i32)
    n97 = Unbundle By Name(w171) -> ("Joystick VS Vision Latch"=w196:bool)
    n98 = Unbundle By Name(w171) -> ("Drive Axes"=w178:dbl[])
    n99 = global read "Robot Global Data.vi" "Robot Mode"() -> (w183:T17)
    n100 = Index Array(array=w170, index #1=2 ("index"), index #2=3 ("index")) -> (element #1=w169:T1, element #2=w168:T1)
    n101 = Bundle By Name(cluster=w171, "Robot Mode"=w183) -> (w197:T25)
    n102 = Index Array(array=w177, index=w194) -> (element=w195:bool)
    n103 = global read "Robot Global Data.vi" "Which Robot?"() -> (w141:T29)
    n104 = Index Array(array=w178, index #1=w179, index #2=w180, index #3=w181, index #4=w182) -> (element #1=w187:dbl, element #2=w188:dbl, element #3=w189:dbl, element #4=w190:dbl)
    n105 = global read "Robot Global Data.vi" "Which Robot?"() -> (w147:T29)
    n106 = Index Array(array=w176, index=w175) -> (element=w173:bool)
    n107 = global read "Robot Global Data.vi" "Right Encoder Val. Initial"() -> (w148:dbl)
    n108 = global read "Robot Global Data.vi" "Left Encoder Val. Initial"() -> (w150:dbl)
    n109 = disable-structure shown="Enabled" {
      disable-tunnel: w195 -> [w382 w389]
      disable-tunnel: w196 -> [_ w387]
      disable-tunnel: w197 -> [_ w385]
      disable-tunnel: [_ w383] -> w174
      frame Disabled {
        n110 = feedback #2() -> (w381:bool)  [unwired: 1 in]
        n111 = feedback-in #2(w382) -> ()
        n112 = Greater?(x=w382, y=w381) -> (0:w380:bool)
        n113 = global write "Robot Global Data.vi" "Driver VS Vision Control"(w380) -> ()
      }
      frame Enabled {
        n114 = feedback #3() -> (w390:bool)  [unwired: 1 in]
        n115 = feedback-in #3(w389) -> ()
        n116 = Greater?(x=w389, y=w390) -> (0:w388:bool)
        n117 = Not(x=w387) -> (.not. x?=w386:bool)
        n118 = Select(t=w386, s=w388, f=w387) -> (s? t:f=w384:bool)
        n119 = global write "Robot Global Data.vi" "Driver VS Vision Control"(w384) -> ()
        n120 = Bundle By Name(cluster=w385, "Joystick VS Vision Latch"=w384) -> (w383:T25)
      }
    }
    n121 = call "Deadband.vi"("Input"=w187) -> ("Output"=w185:dbl)  [unwired: 10 in]
    n122 = call "Deadband.vi"("Input"=w188) -> ("Output"=w186:dbl)  [unwired: 10 in]
    n123 = call "Deadband.vi"("Input"=w189) -> ("Output"=w184:dbl)  [unwired: 10 in]
    n124 = call "Deadband.vi"("Input"=w190) -> ("Output"=w191:dbl)  [unwired: 10 in]
    n125 = call-poly <vilib>:"CTRE_Phoenix_MotorController_Get_Enhanced.vi"("PhoenixMotorControlDevRef"=w169) -> ("Quadrature Position"=w151:i32)  [unwired: 11 in, 3 out]
    n126 = call-poly <vilib>:"CTRE_Phoenix_MotorController_Get_Enhanced.vi"("PhoenixMotorControlDevRef"=w168) -> ("Quadrature Position"=w149:i32)  [unwired: 11 in, 3 out]
    n127 = Negate(x=w186) -> (-x=w192:dbl)
    n128 = Negate(x=w191) -> (-x=w193:dbl)
    n129 = global write "Robot Global Data.vi" "Left Drive Joystick X"(w185) -> ()
    n130 = global write "Robot Global Data.vi" "Right Drive Joystick X"(w184) -> ()
    n131 = case shown="\"Competition Bot\", Default" w141 {
      tunnel: [w213 w215 w217] -> w140
      tunnel: [w212 w214 w216] -> w139
      frame "Competition Bot", Default {
        w212 = 18069  # Change in Encoder
        w213 = 84  # Change in Distance (inches)
      }
      frame "Practice Bot" {
        w214 = 0  # Change in Encoder
        w215 = 0  # Change in Distance (inches)
      }
      frame "Code Bot" {
        w216 = 0  # Change in Encoder
        w217 = 0  # Change in Distance (inches)
      }
    }
    n132 = global write "Robot Global Data.vi" "Right Drive Joystick Y"(w193) -> ()
    n133 = global write "Robot Global Data.vi" "Left Drive Joystick Y"(w192) -> ()
    n134 = case shown="\"Competition Bot\", Default" w147 {
      tunnel: [w219 w221 w223] -> w146
      tunnel: [w218 w220 w222] -> w145
      frame "Competition Bot", Default {
        w218 = 17996  # Change in Encoder
        w219 = 84  # Change in Distance (inches)
      }
      frame "Practice Bot" {
        w220 = 0  # Change in Encoder
        w221 = 0  # Change in Distance (inches)
      }
      frame "Code Bot" {
        w222 = 0  # Change in Encoder
        w223 = 0  # Change in Distance (inches)
      }
    }
    n135 = Subtract(x=w151, y=w150) -> (x-y=w143:dbl)
    n136 = Subtract(x=w149, y=w148) -> (x-y=w137:dbl)
    n137 = Bundle By Name(cluster=w174, "Vision Track Mode Override"=w173) -> (w126:T25)
    n138 = global write "Robot Global Data.vi" "Right Encoder in Enc. Vals"(w137) -> ()
    n139 = global write "Robot Global Data.vi" "Left Encoder in Enc. Vals"(w143) -> ()
    n140 = Divide(x=w140, y=w139) -> (x/y=w136:dbl)
    n141 = Divide(x=w146, y=w145) -> (x/y=w144:dbl)
    n142 = Multiply(x=w144, y=w143) -> (x*y=w142:dbl)
    n143 = Multiply(x=w137, y=w136) -> (x*y=w138:dbl)
    n144 = global write "Robot Global Data.vi" "Left Encoder in Inches"(w142) -> ()
    n145 = global write "Robot Global Data.vi" "Right Encoder in Inches"(w138) -> ()
    n146 = disable-structure shown="Enabled" {
      disable-tunnel: w126 -> [w273 w280]
      frame Disabled {
        n147 = Unbundle By Name(w273) -> ("Drive Button Indexes.RB Button"=w272:i32)
        n148 = Unbundle By Name(w273) -> ("Drive Buttons"=w271:bool[])
        n149 = Unbundle By Name(w273) -> ("T = Motion Profile, F = Percent Output"=w266:bool)
        n150 = Index Array(array=w271, index=w272) -> (element=w269:bool)
        n151 = feedback #4() -> (w270:bool)  [unwired: 1 in]
        n152 = feedback-in #4(w269) -> ()
        n153 = Greater?(x=w269, y=w270) -> (0:w268:bool)
        n154 = Not(x=w266) -> (.not. x?=w267:bool)
        n155 = Select(t=w267, s=w268, f=w266) -> ()  [unwired: 1 out]
      }
      frame Enabled {
        n156 = Unbundle By Name(w280) -> ("Drive Button Indexes.Y Button"=w282:i32)
        n157 = Unbundle By Name(w280) -> ("Drive Buttons"=w281:bool[])
        n158 = global read "Robot Global Data.vi" "Cancel the Motion Profile?"() -> (w274:bool)
        n159 = Index Array(array=w281, index=w282) -> (element=w276:bool)
        n160 = feedback #5() -> (w279:bool)  [unwired: 1 in]
        n161 = feedback-in #5(w276) -> ()
        n162 = Greater?(x=w276, y=w279) -> (0:w278:bool)
        n163 = Not(x=w274) -> (.not. x?=w277:bool)
        n164 = Select(t=w277, s=w278, f=w274) -> (s? t:f=w275:bool)
        n165 = global write "Robot Global Data.vi" "Cancel the Motion Profile?"(w275) -> ()
      }
    }
    n166 = Unbundle By Name(w126) -> ("Drive Button Indexes.RB Button"=w133:i32)
    n167 = Unbundle By Name(w126) -> ("Drive Buttons"=w132:bool[])
    n168 = Index Array(array=w132, index=w133) -> (element=w131:bool)
    n169 = Bundle By Name(cluster=w126, "Arcade Drive?"=w131) -> (w125:T25)
    n170 = call "RIGHT Motion Profile Traj Points Array.vi"("Read = false, Write = true"=FALSE) -> ("traj. points array out"=w152:dbl[][])  [unwired: 10 in]
    "Right Traj. Pts Array" <- w152
    n171 = call "LEFT Motion Profile Traj Points Array.vi"("Read = false, Write = true"=FALSE) -> ("traj. points array out"=w159:dbl[][])  [unwired: 10 in]
    "Left Traj. Pts Array" <- w159
    n172 = for {
      N -> [w237]
      tunnel: w152 -> [w243] mode=indexing
      tunnel: [w233] -> w158 mode=indexing
      i -> [w236]
      w242 = 0.0 ("Arbitrary Feed Forward")
      # "Convert profile units to talon units"
      n173 = Decrement(x=w237) -> (x-1=w238:i32)
      n174 = Equal?(x=w238, y=w236) -> (x = y?=w239:bool)
      n175 = Equal To 0?(x=w236) -> (x = 0?=w235:bool)
      n176 = Index Array(array=w243) -> (element #1=w231:dbl, element #2=w225:dbl, element #3=w232:dbl)  [unwired: 3 in]
      n177 = Multiply(x=4096.0, y=w225) -> (x*y=w227:dbl)
      n178 = Multiply(x=4096.0, y=w231) -> (x*y=w229:dbl)
      n179 = Divide(x=w227, y=10.0) -> (x/y=w224:dbl)
      n180 = Bundle By Name(cluster=T28 {"Position"=0.0, "Velocity"=0.0, "Arbitrary Feed Forward"=0.0, "Auxiliary Position"=0.0, "Auxiliary Velocity"=0.0, "Auxiliary Arbitrary Feed Forward"=0.0, "Profile Slot Select"=0, "Auxiliary Profile Slot Select"=0, "isLastPoint?"=FALSE, "Zero Position?"=FALSE, "durationMs"=0, "Use Aux PID?"=FALSE} ("Trajectory Point"), "Position"=w229, "Velocity"=w224, "Arbitrary Feed Forward"=w242, "Auxiliary Position"=w242, "Auxiliary Velocity"=w242, "Auxiliary Arbitrary Feed Forward"=w242, "Profile Slot Select"=0, "Auxiliary Profile Slot Select"=1, "isLastPoint?"=w239, "Zero Position?"=w235, "durationMs"=w232, "Use Aux PID?"=FALSE) -> (w233:T28)
    }
    n181 = for {
      N -> [w258]
      tunnel: w159 -> [w264] mode=indexing
      tunnel: [w254] -> w165 mode=indexing
      i -> [w257]
      w263 = 0.0 ("Arbitrary Feed Forward")
      # "Convert profile units to talon units"
      n182 = Decrement(x=w258) -> (x-1=w259:i32)
      n183 = Equal?(x=w259, y=w257) -> (x = y?=w260:bool)
      n184 = Equal To 0?(x=w257) -> (x = 0?=w256:bool)
      n185 = Index Array(array=w264) -> (element #1=w252:dbl, element #2=w246:dbl, element #3=w253:dbl)  [unwired: 3 in]
      n186 = Multiply(x=4096.0, y=w246) -> (x*y=w248:dbl)
      n187 = Multiply(x=4096.0, y=w252) -> (x*y=w250:dbl)
      n188 = Divide(x=w248, y=10.0) -> (x/y=w245:dbl)
      n189 = Bundle By Name(cluster=T28 {"Position"=0.0, "Velocity"=0.0, "Arbitrary Feed Forward"=0.0, "Auxiliary Position"=0.0, "Auxiliary Velocity"=0.0, "Auxiliary Arbitrary Feed Forward"=0.0, "Profile Slot Select"=0, "Auxiliary Profile Slot Select"=0, "isLastPoint?"=FALSE, "Zero Position?"=FALSE, "durationMs"=0, "Use Aux PID?"=FALSE} ("Trajectory Point"), "Position"=w250, "Velocity"=w245, "Arbitrary Feed Forward"=w263, "Auxiliary Position"=w263, "Auxiliary Velocity"=w263, "Auxiliary Arbitrary Feed Forward"=w263, "Profile Slot Select"=0, "Auxiliary Profile Slot Select"=1, "isLastPoint?"=w260, "Zero Position?"=w256, "durationMs"=w253, "Use Aux PID?"=FALSE) -> (w254:T28)
    }
    n190 = call <vilib>:"CTRE_Phoenix_MotorControl_BufferedTrajectoryPointStream_Open.vi"() -> ("BufferedTrajectoryPointStream_DevRef"=w157:T30)  [unwired: 10 in, 1 out]
    n191 = call <vilib>:"CTRE_Phoenix_MotorControl_BufferedTrajectoryPointStream_Open.vi"() -> ("BufferedTrajectoryPointStream_DevRef"=w164:T30)  [unwired: 10 in, 1 out]
    n192 = call-poly <vilib>:"CTRE_Phoenix_MotorControl_BufferedTrajectoryPointStream_Write.vi"("Motion Profile Trajectory Point Array"=w158, "BufferedTrajectoryPointStream_DevRef"=w157) -> ("error out"=w155:errorcluster, "BufferedTrajectoryPointStream_DevRef"=w156:T30)  [unwired: 8 in]
    n193 = call-poly <vilib>:"CTRE_Phoenix_MotorControl_BufferedTrajectoryPointStream_Write.vi"("Motion Profile Trajectory Point Array"=w165, "BufferedTrajectoryPointStream_DevRef"=w164) -> ("error out"=w162:errorcluster, "BufferedTrajectoryPointStream_DevRef"=w163:T30)  [unwired: 8 in]
    n194 = call <vilib>:"CTRE_Phoenix_MotorControl_BufferedTrajectoryPointStream_SetDeviceReference.vi"("error in (no error)"=w155, "refnum name"="right_mpStream", "BufferedTrajectoryPointStream_DevRef"=w156) -> ()  [unwired: 7 in, 2 out]
    n195 = call <vilib>:"CTRE_Phoenix_MotorControl_BufferedTrajectoryPointStream_SetDeviceReference.vi"("error in (no error)"=w162, "refnum name"="left_mpStream", "BufferedTrajectoryPointStream_DevRef"=w163) -> ()  [unwired: 7 in, 2 out]
    n196 = Unbundle By Name(w125) -> ("T = Motion Profile, F = Percent Output"=w130:bool)
    n197 = Unbundle By Name(w125) -> ("Start Motion Profile?"=w124:bool)
    n198 = case shown="False" w130 {
      tunnel: [w284 w376] -> w210
      tunnel: w125 -> [w283 w377]
      tunnel: w124 -> [_ w375]
      frame False {
        n199 = disable-structure shown="Enabled" {
          disable-tunnel: [w300 w320] -> w284
          disable-tunnel: w283 -> [w292 w306]
          frame Enabled {
            # "Vision and Joystick Control for Drive Train"
            # "for ease of testing\nfor programmers"
            # "1 = force off\n3 = force on"
            # "0 = vision processor\n1 = driver camera settings"
            n200 = Unbundle By Name(w292) -> ("Joystick VS Vision Latch"=w296:bool)
            n201 = Unbundle By Name(w292) -> ("Vision Track Mode Override"=w288:bool)
            n202 = Select(t=3, s=w296, f=1) -> (s? t:f=w287:i32)
            n203 = Select(t=0, s=w296, f=1) -> (s? t:f=w291:i32)
            n204 = Select(t=3, s=w288, f=w287) -> (s? t:f=w286:i32)
            n205 = Select(t=0, s=w288, f=w291) -> (s? t:f=w289:i32)
            n206 = case shown="True" w296 {
              tunnel: w292 -> [w301 w303]
              tunnel: [w301 w304] -> w300
              frame False {
                n207 = Unbundle By Name(w301) -> ("Arcade Drive?"=w302:bool)
                n208 = call "Joystick Drive Control.vi"("Arcade Drive?"=w302, "Cluster In"=w301) -> ()  [unwired: 10 in]
              }
              frame True {
                n209 = call "Vision Tracking Drive Control.vi"("Cluster In"=w303) -> ("Cluster Out"=w304:T25)  [unwired: 10 in]
              }
            }
            n210 = call-poly <vilib>:"NT Write Value.vi"("Numeric"=w289, "Name"="/limelight/camMode") -> ()  [unwired: 9 in, 1 out]
            n211 = call-poly <vilib>:"NT Write Value.vi"("Numeric"=w286, "Name"="/limelight/ledMode") -> ()  [unwired: 9 in, 1 out]
          }
          frame Disabled {
            n212 = call-poly <vilib>:"NT Read Value.vi"("Name"="/limelight/tx") -> ("Numeric"=w314:dbl)  [unwired: 9 in, 1 out]
            n213 = call-poly <vilib>:"NT Read Value.vi"("Name"="/limelight/ty") -> ("Numeric"=w313:dbl)  [unwired: 9 in, 1 out]
            n214 = call-poly <vilib>:"NT Read Value.vi"("Name"="/limelight/ta") -> ("Numeric"=w312:dbl)  [unwired: 9 in, 1 out]
            n215 = call-poly <vilib>:"NT Read Value.vi"("Name"="/limelight/ts") -> ("Numeric"=w311:dbl)  [unwired: 9 in, 1 out]
            n216 = call-poly <vilib>:"NT Read Value.vi"("Name"="/limelight/tshort") -> ("Numeric"=w308:dbl)  [unwired: 9 in, 1 out]
            n217 = call-poly <vilib>:"NT Read Value.vi"("Name"="/limelight/tlong") -> ("Numeric"=w307:dbl)  [unwired: 9 in, 1 out]
            n218 = Bundle By Name(cluster=w306, "limelight.offsetAngle H"=w314, "limelight.offsetAngle V"=w313, "limelight.area"=w312, "limelight.skew"=w311, "limelight.shortest side (pxls)"=w308, "limelight.longest side (pxls)"=w307) -> (w305:T25)
            n219 = Unbundle By Name(w305) -> ("Vision States"=w322:T19)
            n220 = case shown="\"Ready\", Default" w322 {
              tunnel: [w323 w338 w356] -> w321
              tunnel: w305 -> [w323 w338 w356]
              tunnel: [w332 w339 w352] -> w319
              frame "Ready", Default {
                # "should have created a \nboolean in the cluster \ninstead of just pulling\nthe A button"
                # "the Ys of the drive joysticks are \ninverted by default"
                n221 = Unbundle By Name(w323) -> ("Drive Button Indexes.A Button"=w337:i32)
                n222 = Unbundle By Name(w323) -> ("Drive Buttons"=w336:bool[])
                n223 = Unbundle By Name(w323) -> ("Drive Motors"=w331:T11, "Drive Axes"=w330:dbl[], "Drive Axes Indexes.Left Y"=w329:i32, "Drive Axes Indexes.Right Y"=w328:i32)
                n224 = Index Array(array=w336, index=w337) -> (element=w335:bool)
                n225 = Index Array(array=w330, index #1=w329, index #2=w328) -> (element #1=w327:dbl, element #2=w326:dbl)
                n226 = Negate(x=w327) -> (-x=w324:dbl)
                n227 = Negate(x=w326) -> (-x=w325:dbl)
                n228 = Select(t=Vision_States."Forward Until Target at Edge" ("Vision States"), s=w335, f=Vision_States."Ready" ("Vision States")) -> (s? t:f=w332:T19)
                n229 = call <vilib>:"WPI_RobotDriveTankDrive.vi"("Right axis value"=w325, "Left axis value"=w324, "RobotDriveDevRef"=w331) -> ()  [unwired: 6 in, 3 out]
              }
              frame "Forward Until Target at Edge" {
                n230 = Unbundle By Name(w338) -> ("limelight.offsetAngle H"=w343:dbl)
                n231 = Less?(x=w343, y=-26) -> (x < y?=w341:bool)
                n232 = Greater?(x=w343, y=14) -> (0:w342:bool)
                n233 = Or(x=w342, y=w341) -> (x .or. y?=w340:bool)
                n234 = case shown="False" w340 {
                  tunnel: [Vision_States."Forward Until Target at Edge" ("Vision States") Vision_States."Vision Track" ("Vision States")] -> w339
                  tunnel: w338 -> [w349 _]
                  frame False {
                    w347 = 0.35
                    n235 = Unbundle By Name(w349) -> ("Drive Motors"=w348:T11)
                    n236 = call <vilib>:"WPI_RobotDriveTankDrive.vi"("Right axis value"=w347, "Left axis value"=w347, "RobotDriveDevRef"=w348) -> ()  [unwired: 6 in, 3 out]
                  }
                  frame True {
                  }
                }
              }
              frame "Vision Track" {
                w359 = 0.5 ("t")
                w358 = 1.5
                # "this is the target area for\nwhen to stop driving \ntoward target (10 here \nwould means 10% of \nlimelight feed)"
                # "Hori. offset scaled down to\nbe a reasonable drive speed\ncoefficient (e.g. if this number\nis 0.01, 10deg offset to the \nleft would make right train \nrun at 110% and left train \nat 90%)"
                # "0deg offset = speed \nadjustment coefficient of 1"
                n237 = Unbundle By Name(w356) -> ("limelight.area"=w364:dbl, "limelight.offsetAngle H"=w372:dbl)
                n238 = Multiply(x=w372, y=0.03) -> (x*y=w361:dbl)
                n239 = Unbundle By Name(w356) -> ("Drive Motors"=w357:T11)
                n240 = Add(x=1.0, y=w361) -> (x+y=w367:dbl)
                n241 = Subtract(x=1.0, y=w361) -> (x-y=w360:dbl)
                n242 = Less?(x=w364, y=w358) -> (x < y?=w355:bool)
                n243 = Less?(x=w364, y=w358) -> (x < y?=w368:bool)
                n244 = Select(t=w359, s=w355, f=0.0) -> (s? t:f=w373:dbl)
                n245 = Select(t=w359, s=w368, f=0.0) -> (s? t:f=w365:dbl)
                n246 = Multiply(x=w373, y=w367) -> (x*y=w370:dbl)
                n247 = Multiply(x=w360, y=w365) -> (x*y=w363:dbl)
                n248 = Not(x=w355) -> (.not. x?=w351:bool)
                n249 = call <vilib>:"WPI_RobotDriveTankDrive.vi"("Right axis value"=w363, "Left axis value"=w370, "RobotDriveDevRef"=w357) -> ()  [unwired: 6 in, 3 out]
                n250 = Select(t=Vision_States."Ready" ("Vision States"), s=w351, f=Vision_States."Vision Track" ("Vision States")) -> (s? t:f=w352:T19)
              }
            }
            n251 = Bundle By Name(cluster=w321, "Vision States"=w319) -> (w320:T25)
          }
        }
      }
      frame True {
        # "left MP will control when the motion profile ends"
        # "Motion Profile Control for Drive Train"
        n252 = call "Motion Profile Left Drive Control.vi"("Start Motion Profile?"=w375, "Cluster In"=w377) -> ("Cluster Out"=w376:T25)  [unwired: 9 in]
        n253 = call "Motion Profile Right Drive Control.vi"("Start Motion Profile?"=w375, "Cluster In"=w377) -> ()  [unwired: 9 in, 1 out]
      }
    }
  }
  n254 = disable-structure shown="Disabled" {
    disable-tunnel: w84 -> [w507 _]
    frame Disabled {
      # "Collector Angle and Retainer Motor"
      # "Collector Pneumatics"
      # "Defining Global Data Values and Some Cluster Values"
      # "Defining Array Values for Joysticks"
      n255 = while {
        shift-right: [w511] -> _
        shift-left: w507 -> [w557]
        stop <- FALSE stop-if-true
        # "this chunk of code \ncontrols the wanted\nangle of the collector\nusing a joystick and\n2 angle presets"
        # "use this to scale the rate at which the\nwanted angle changes based on the joystick"
        # "we use this to set the\n\"0\" of the encoder to be \nwherever it is when the code\nis run (or the robot is turned\non in the case of \nhard-deployed code)"
        # "this chunk of code \nconverts the encoder\n values into angles"
        n256 = Unbundle By Name(w557) -> ("DriveJoystickDevRef"=w568:T9)
        n257 = Unbundle By Name(w557) -> ("AuxJoystickDevRef"=w567:T9)
        n258 = Unbundle By Name(w557) -> ("Robot Mode"=w566:T17)
        n259 = Wait (ms)(milliseconds to wait=u32 50) -> ()  [unwired: 1 out]
        n260 = call <vilib>:"WPI_JoystickGetValues.vi"("JoystickDevRef"=w567) -> ("Buttons"=w559:bool[], "Axes"=w560:dbl[], "JoystickDevRef"=w561:T9, "POVs"=w558:i16[])  [unwired: 6 in, 1 out]
        n261 = call <vilib>:"WPI_JoystickGetValues.vi"("JoystickDevRef"=w568) -> ("Buttons"=w563:bool[], "Axes"=w565:dbl[], "JoystickDevRef"=w564:T9, "POVs"=w562:i16[])  [unwired: 6 in, 1 out]
        n262 = case shown="\"Teleop Enabled\"" w566 {
          tunnel: w557 -> [w786 w796 w797 w798 w808 w809 w810 w820 w821]
          tunnel: [w786 w787 w797 w799 w808 w809 w810 w811 w821] -> w534
          tunnel: w565 -> [_ w795 _ w806 _ _ _ w818 _]
          tunnel: w564 -> [_ w794 _ w807 _ _ _ w819 _]
          tunnel: w563 -> [_ w793 _ w805 _ _ _ w817 _]
          tunnel: w562 -> [_ w792 _ w804 _ _ _ w816 _]
          tunnel: w561 -> [_ w791 _ w803 _ _ _ w815 _]
          tunnel: w560 -> [_ w790 _ w802 _ _ _ w814 _]
          tunnel: w559 -> [_ w789 _ w801 _ _ _ w813 _]
          tunnel: w558 -> [_ w788 _ w800 _ _ _ w812 _]
          frame "Autonomous Disabled", Default {
          }
          frame "Autonomous Enabled" {
            n263 = Bundle By Name(cluster=w796, "DriveJoystickDevRef"=w794, "Drive Axes"=w795, "Drive Buttons"=w793, "Drive POVs"=w792, "AuxJoystickDevRef"=w791, "Aux Axes"=w790, "Aux Buttons"=w789, "Aux POVs"=w788) -> (w787:T26)
          }
          frame "Teleop Disabled" {
          }
          frame "Teleop Enabled" {
            n264 = Bundle By Name(cluster=w798, "DriveJoystickDevRef"=w807, "Drive Axes"=w806, "Drive Buttons"=w805, "Drive POVs"=w804, "AuxJoystickDevRef"=w803, "Aux Axes"=w802, "Aux Buttons"=w801, "Aux POVs"=w800) -> (w799:T26)
          }
          frame "Disconnected" {
          }
          frame "Finish" {
          }
          frame "Test Disabled" {
          }
          frame "Test Enabled" {
            n265 = Bundle By Name(cluster=w820, "DriveJoystickDevRef"=w819, "Drive Axes"=w818, "Drive Buttons"=w817, "Drive POVs"=w816, "AuxJoystickDevRef"=w815, "Aux Axes"=w814, "Aux Buttons"=w813, "Aux POVs"=w812) -> (w811:T26)
          }
          frame "Emergency Stopped" {
          }
        }
        n266 = Unbundle By Name(w534) -> ("Aux Button Indexes.RB Button"=w532:i32)
        n267 = Unbundle By Name(w534) -> ("Aux Button Indexes.RT Button"=w531:i32)
        n268 = Unbundle By Name(w534) -> ("Aux Joystick Indexes.Right Y"=w541:i32)
        n269 = Unbundle By Name(w534) -> ("Aux Button Indexes.LT Button"=w555:i32)
        n270 = Unbundle By Name(w534) -> ("Aux Axes"=w542:dbl[])
        n271 = Unbundle By Name(w534) -> ("Aux Buttons"=w533:bool[])
        n272 = Unbundle By Name(w534) -> ("Aux Buttons"=w554:bool[])
        n273 = Unbundle By Name(w534) -> ("Hatch Collector Wanted Angle"=w539:dbl)
        n274 = Unbundle By Name(w534) -> ("Hatch Retainer Move Up/Down"=w551:bool)
        n275 = Unbundle By Name(w534) -> ("HatchCollectorMotorDevRef"=w548:T1)
        n276 = global read "Robot Global Data.vi" "Hatch Encoder Start Value"() -> (w543:dbl)
        n277 = global read "Robot Global Data.vi" "Robot Mode"() -> (w556:T17)
        n278 = global read "Robot Global Data.vi" "Which Robot?"() -> (w519:T29)
        n279 = Bundle By Name(cluster=w534, "Robot Mode"=w556) -> (w553:T26)
        n280 = call-poly <vilib>:"CTRE_Phoenix_MotorController_Get_Enhanced.vi"("PhoenixMotorControlDevRef"=w548) -> ("Quadrature Position"=w546:i32)  [unwired: 11 in, 3 out]
        n281 = Index Array(array=w542, index=w541) -> (element=w525:dbl)
        n282 = Index Array(array=w554, index=w555) -> (element=w552:bool)
        n283 = Index Array(array=w533, index #1=w532, index #2=w531) -> (element #1=w528:bool, element #2=w529:bool)
        n284 = call "Deadband.vi"("Input"=w525) -> ("Output"=w523:dbl)  [unwired: 10 in]
        n285 = disable-structure shown="Enabled" {
          disable-tunnel: w552 -> [w741 w745]
          disable-tunnel: w551 -> [w738 _]
          disable-tunnel: [w737 w744] -> w550
          frame Disabled {
            n286 = feedback #6() -> (w742:bool)  [unwired: 1 in]
            n287 = feedback-in #6(w741) -> ()
            n288 = Greater?(x=w741, y=w742) -> (0:w740:bool)
            n289 = Not(x=w738) -> (.not. x?=w739:bool)
            n290 = Select(t=w739, s=w740, f=w738) -> (s? t:f=w737:bool)
          }
          frame Enabled {
            n291 = feedback #7() -> (w743:bool)  [unwired: 1 in]
            n292 = feedback-in #7(w745) -> ()
            n293 = Greater?(x=w745, y=w743) -> (0:w744:bool)
          }
        }
        n294 = case shown="\"Competition Bot\", Default" w519 {
          tunnel: [w761 w770 w779] -> w547
          tunnel: w546 -> [w759 w769 w778]
          tunnel: w543 -> [w760 w768 w777]
          frame "Competition Bot", Default {
            # "range of \ndegrees"
            # "enc. val at\n\"max out\"\ndeg IRL"
            # "enc. val at\n\"max in\"\ndeg IRL"
            n295 = Subtract(x=w759, y=w760) -> (x-y=w762:dbl)
            n296 = Subtract(x=1047.0, y=46.0) -> (x-y=w766:dbl)
            n297 = Divide(x=97.0, y=w766) -> (x/y=w764:dbl)
            n298 = Multiply(x=w764, y=w762) -> (x*y=w761:dbl)
          }
          frame "Practice Bot" {
            # "range of \ndegrees"
            # "enc. val at\n\"max out\"\ndeg IRL"
            # "enc. val at\n\"max in\"\ndeg IRL"
            n299 = Subtract(x=w769, y=w768) -> (x-y=w771:dbl)
            n300 = Subtract(x=1050.0, y=34.0) -> (x-y=w775:dbl)
            n301 = Divide(x=90.0, y=w775) -> (x/y=w773:dbl)
            n302 = Multiply(x=w773, y=w771) -> (x*y=w770:dbl)
          }
          frame "Code Bot" {
            # "range of \ndegrees"
            # "enc. val at\n\"max out\"\ndeg IRL"
            # "enc. val at\n\"max in\"\ndeg IRL"
            n303 = Subtract(x=w778, y=w777) -> (x-y=w780:dbl)
            n304 = Subtract(x=1050.0, y=34.0) -> (x-y=w784:dbl)
            n305 = Divide(x=90.0, y=w784) -> (x/y=w782:dbl)
            n306 = Multiply(x=w782, y=w780) -> (x*y=w779:dbl)
          }
        }
        n307 = Add(x=w539, y=w523) -> (x+y=w538:dbl)
        n308 = Or(x=w528, y=w529) -> (x .or. y?=w530:bool)
        n309 = Multiply(x=1.0, y=w538) -> (x*y=w535:dbl)
        n310 = case shown="True" w530 {
          tunnel: [w754 w755] -> w536
          tunnel: w535 -> [w754 _]
          tunnel: w528 -> [_ w756]
          frame False {
            # "neither \npreset,\nJS controls\nwanted angle"
          }
          frame True {
            n311 = case shown="True" w756 {
              tunnel: [80.0 7.0] -> w755
              frame False {
                # "preset \nfor \nhovering\nto use \ndustpan"
              }
              frame True {
                # "preset\nfor \nvertical"
              }
            }
          }
        }
        n312 = global read "Robot Global Data.vi" "Which Robot?"() -> (w518:T29)
        n313 = case shown="\"Competition Bot\", Default" w518 {
          tunnel: [97.0 99.0 90.0] -> w517
          frame "Competition Bot", Default {
            # "max deg"
          }
          frame "Practice Bot" {
            # "max deg"
          }
          frame "Code Bot" {
            # "max deg"
          }
        }
        n314 = In Range and Coerce(upper limit=w517, x=w536, lower limit=0.0) -> (coerced(x)=w527:dbl)  [unwired: 1 out]
        n315 = Bundle By Name(cluster=w553, "Hatch Retainer Move Up/Down"=w550) -> (w549:T26)
        n316 = Bundle By Name(cluster=w549, "Hatch Collector Actual Angle"=w547) -> (w540:T26)
        n317 = Bundle By Name(cluster=w540, "Hatch Collector Wanted Angle"=w527) -> (w512:T26)
        n318 = disable-structure shown="Enabled" {
          disable-tunnel: [w661 w684] -> w513
          disable-tunnel: w512 -> [w659 w694]
          disable-tunnel: w512 -> [w658 w687]
          frame Disabled {
            # "only let kickers kick\nif the hatch retainer\nis fully down"
            # "if kick button was just pressed, go\ndown. Otherwise, keep the states\nas they are"
            n319 = Unbundle By Name(w658) -> ("KickerSolenoidDevRef"=w676:T6)
            n320 = Unbundle By Name(w658) -> ("Hatch Retainer States"=w663:T14)
            n321 = Unbundle By Name(w658) -> ("Aux Button Indexes.LB Button"=w674:i32)
            n322 = Unbundle By Name(w658) -> ("Aux Buttons"=w675:bool[])
            n323 = global read "Robot Global Data.vi" "Kick Hatch in Auto"() -> (w669:bool)
            n324 = case shown="\"Fully Down (not retained)\", Default" w663 {
              tunnel: [TRUE FALSE FALSE FALSE] -> w667
              frame "Fully Down (not retained)", Default {
              }
              frame "Going Up" {
              }
              frame "Fully Up (retained)" {
              }
              frame "Going Down" {
              }
            }
            n325 = Index Array(array=w675, index=w674) -> (element=w670:bool)
            n326 = Or(x=w670, y=w669) -> (x .or. y?=w665:bool)
            n327 = And(x=w665, y=w667) -> (x .and. y?=w668:bool)
            n328 = feedback #8() -> (w666:bool)  [unwired: 1 in]
            n329 = feedback-in #8(w665) -> ()
            n330 = Select(t=WPI_SolenoidValue."On" ("Value"), s=w668, f=WPI_SolenoidValue."Off" ("Value")) -> (s? t:f=w671:T31)
            n331 = Greater?(x=w665, y=w666) -> (0:w664:bool)
            n332 = call-poly <vilib>:"WPI_SolenoidSet.vi"("Value"=w671, "SolenoidDevRef"=w676) -> ()  [unwired: 8 in, 2 out]
            n333 = Select(t=Hatch_Retainer_States."Going Down" ("Hatch Retainer States"), s=w664, f=w663) -> (s? t:f=w662:T14)
            n334 = Bundle By Name(cluster=w659, "Hatch Retainer States"=w662) -> (w661:T26)
          }
          frame Enabled {
            n335 = Unbundle By Name(w687) -> ("Aux Button Indexes.LB Button"=w692:i32)
            n336 = Unbundle By Name(w687) -> ("Hatch Kicking States"=w682:T12)
            n337 = Unbundle By Name(w687) -> ("Aux Buttons"=w693:bool[])
            n338 = Unbundle By Name(w687) -> ("Hatch Retainer States"=w686:T14)
            n339 = Unbundle By Name(w687) -> ("KickerSolenoidDevRef"=w691:T6)
            n340 = feedback #9() -> (w681:T12)  [unwired: 1 in]
            n341 = feedback-in #9(w682) -> ()
            n342 = Index Array(array=w693, index=w692) -> (element=w688:bool)
            n343 = case shown="\"Kick Hatch\"" w682 {
              selector: w682 -> [_ _ w719]
              tunnel: [WPI_SolenoidValue."Off" ("Value") WPI_SolenoidValue."Off" ("Value") w716] -> w690
              tunnel: [w696 w703 w720] -> w689
              tunnel: w688 -> [w699 _ _]
              tunnel: w686 -> [w695 w701 w724]
              tunnel: [w695 w704 w724] -> w683
              tunnel: w681 -> [_ _ w717]
              frame "Ready", Default {
                n344 = Select(t=Hatch_Kicking_States."Stop Retaining Hatch" ("Hatch Kicking States"), s=w699, f=Hatch_Kicking_States."Ready" ("Hatch Kicking States")) -> (s? t:f=w696:T12)
              }
              frame "Stop Retaining Hatch" {
                n345 = Equal?(x=Hatch_Retainer_States."Fully Down (not retained)" ("Hatch Retainer States"), y=w701) -> (x = y?=w705:bool)
                n346 = case shown="False" w705 {
                  tunnel: [Hatch_Retainer_States."Going Down" ("Hatch Retainer States") Hatch_Retainer_States."Fully Down (not retained)" ("Hatch Retainer States")] -> w704
                  tunnel: [Hatch_Kicking_States."Stop Retaining Hatch" ("Hatch Kicking States") Hatch_Kicking_States."Kick Hatch" ("Hatch Kicking States")] -> w703
                  frame False {
                  }
                  frame True {
                  }
                }
              }
              frame "Kick Hatch" {
                # "if previous state\nis not the same \nas the current, we\njust entered \"kick\nhatch\" and \nshould reset our\ntimer"
                n347 = Not Equal?(x=w719, y=w717) -> (x != y?=w718:bool)
                n348 = call "Elapsed Time"("Reset"=w718) -> ("Elapsed Time (s)"=w714:dbl)  [unwired: 11 in, 7 out]
                n349 = Greater Or Equal?(x=w714, y=1.5) -> (x >= y?=w723:bool)
                n350 = Less Or Equal?(x=w714, y=0.5) -> (x <= y?=w715:bool)
                n351 = Select(t=WPI_SolenoidValue."On" ("Value"), s=w715, f=WPI_SolenoidValue."Off" ("Value")) -> (s? t:f=w716:T31)
                n352 = Select(t=Hatch_Kicking_States."Ready" ("Hatch Kicking States"), s=w723, f=Hatch_Kicking_States."Kick Hatch" ("Hatch Kicking States")) -> (s? t:f=w720:T12)
              }
            }
            n353 = Bundle By Name(cluster=w694, "Hatch Kicking States"=w689) -> (w685:T26)
            n354 = Bundle By Name(cluster=w685, "Hatch Retainer States"=w683) -> (w684:T26)
            n355 = call-poly <vilib>:"WPI_SolenoidSet.vi"("Value"=w690, "SolenoidDevRef"=w691) -> ()  [unwired: 8 in, 2 out]
          }
        }
        n356 = Unbundle By Name(w512) -> ("RetainerSolenoidDevRef"=w510:T6)
        n357 = disable-structure shown="Disabled" {
          disable-tunnel: w512 -> [w746 _]
          frame Disabled {
            n358 = Unbundle By Name(w746) -> ("Aux Button Indexes.B Button"=w753:i32)
            n359 = Unbundle By Name(w746) -> ("LifterSolenoidDevRef"=w747:T6)
            n360 = Unbundle By Name(w746) -> ("Aux Buttons"=w752:bool[])
            n361 = Index Array(array=w752, index=w753) -> (element=w749:bool)
            n362 = Select(t=WPI_SolenoidValue."On" ("Value"), s=w749, f=WPI_SolenoidValue."Off" ("Value")) -> (s? t:f=w748:T31)
            n363 = call-poly <vilib>:"WPI_SolenoidSet.vi"("Value"=w748, "SolenoidDevRef"=w747) -> ()  [unwired: 8 in, 2 out]
          }
          frame Enabled {
          }
        }
        n364 = Unbundle By Name(w512) -> ("Hatch Retainer States"=w509:T14)
        n365 = case shown="\"Going Down\"" w509 {
          tunnel: [WPI_SolenoidValue."Off" ("Value") WPI_SolenoidValue."On" ("Value") WPI_SolenoidValue."On" ("Value") WPI_SolenoidValue."Off" ("Value")] -> w508
          frame "Fully Down (not retained)", Default {
          }
          frame "Going Up" {
          }
          frame "Fully Up (retained)" {
          }
          frame "Going Down" {
          }
        }
        n366 = call-poly <vilib>:"WPI_SolenoidSet.vi"("Value"=w508, "SolenoidDevRef"=w510) -> ()  [unwired: 8 in, 2 out]
        n367 = disable-structure shown="Enabled" {
          disable-tunnel: [w581 w626] -> w524
          disable-tunnel: w513 -> [w575 w625]
          frame Disabled {
            n368 = disable-structure shown="Enabled" {
              disable-tunnel: [w585 TRUE] -> w578
              disable-tunnel: [w584 TRUE] -> w577
              disable-tunnel: w575 -> [w583 _]
              frame Disabled {
                n369 = Unbundle By Name(w583) -> ("BottomRetainerSwitchDevRef"=w587:T8)
                n370 = Unbundle By Name(w583) -> ("TopRetainerSwitchDevRef"=w589:T8)
                n371 = call <vilib>:"WPI_DigitalInputGetValue.vi"("DigitalInputDevRef"=w589) -> ("Value"=w588:bool)  [unwired: 8 in, 2 out]
                n372 = call <vilib>:"WPI_DigitalInputGetValue.vi"("DigitalInputDevRef"=w587) -> ("Value"=w586:bool)  [unwired: 8 in, 2 out]
                n373 = Not(x=w586) -> (.not. x?=w584:bool)
                n374 = Not(x=w588) -> (.not. x?=w585:bool)
              }
              frame Enabled {
                # "since we aren't using the limit\nswitches now, this acts like they're\nclicked so we don't have to rewrite\neverything"
              }
            }
            n375 = Unbundle By Name(w575) -> ("Hatch Retainer States"=w582:T14)
            n376 = Unbundle By Name(w575) -> ("HatchRetainerMotorDevRef"=w579:T1)
            n377 = Unbundle By Name(w575) -> ("Hatch Retainer Move Up/Down"=w580:bool)
            n378 = case shown="\"Going Down\"" w582 {
              tunnel: [w595 w600 w614 w619] -> w581
              tunnel: w580 -> [w598 _ w615 _]
              tunnel: w578 -> [_ w602 _ _]
              tunnel: w577 -> [_ _ _ w618]
              tunnel: w579 -> [w592 w601 w610 w617]
              tunnel: 0.2 ("Output") -> [_ w599 _ w616]
              frame "Fully Down (not retained)", Default {
                w594 = T33 0 items=["PercentOutput"=0, "Position"=1, "Velocity"=2, "Current"=3, "Follower"=5, "MotionProfile"=6, "MotionMagic"=7, "MotionProfileArc"=10, "Disabled"=15] ("Control Mode")
                n379 = call <vilib>:"CTRE_Phoenix_MotorControl_Set.vi"("Output"=0.0, "Control Mode"=w594, "PhoenixMotorControlDevRef"=w592) -> ()  [unwired: 7 in, 2 out]
                n380 = Select(t=Hatch_Retainer_States."Going Up" ("Hatch Retainer States"), s=w598, f=Hatch_Retainer_States."Fully Down (not retained)" ("Hatch Retainer States")) -> (s? t:f=w595:T14)
              }
              frame "Going Up" {
                n381 = case shown="True" w602 {
                  tunnel: w601 -> [w607 _]
                  tunnel: [Hatch_Retainer_States."Going Up" ("Hatch Retainer States") Hatch_Retainer_States."Fully Up (retained)" ("Hatch Retainer States")] -> w600
                  tunnel: w599 -> [w604 _]
                  frame False {
                    w605 = T33 0 items=["PercentOutput"=0, "Position"=1, "Velocity"=2, "Current"=3, "Follower"=5, "MotionProfile"=6, "MotionMagic"=7, "MotionProfileArc"=10, "Disabled"=15] ("Control Mode")
                    n382 = Negate(x=w604) -> (-x=w603:dbl)
                    n383 = call <vilib>:"CTRE_Phoenix_MotorControl_Set.vi"("Output"=w603, "Control Mode"=w605, "PhoenixMotorControlDevRef"=w607) -> ()  [unwired: 7 in, 2 out]
                  }
                  frame True {
                  }
                }
              }
              frame "Fully Up (retained)" {
                w611 = T33 0 items=["PercentOutput"=0, "Position"=1, "Velocity"=2, "Current"=3, "Follower"=5, "MotionProfile"=6, "MotionMagic"=7, "MotionProfileArc"=10, "Disabled"=15] ("Control Mode")
                n384 = call <vilib>:"CTRE_Phoenix_MotorControl_Set.vi"("Output"=0.0, "Control Mode"=w611, "PhoenixMotorControlDevRef"=w610) -> ()  [unwired: 7 in, 2 out]
                n385 = Select(t=Hatch_Retainer_States."Going Down" ("Hatch Retainer States"), s=w615, f=Hatch_Retainer_States."Fully Up (retained)" ("Hatch Retainer States")) -> (s? t:f=w614:T14)
              }
              frame "Going Down" {
                n386 = case shown="True" w618 {
                  tunnel: [Hatch_Retainer_States."Going Down" ("Hatch Retainer States") Hatch_Retainer_States."Fully Down (not retained)" ("Hatch Retainer States")] -> w619
                  tunnel: w617 -> [w622 _]
                  tunnel: w616 -> [w620 _]
                  frame False {
                    w621 = T33 0 items=["PercentOutput"=0, "Position"=1, "Velocity"=2, "Current"=3, "Follower"=5, "MotionProfile"=6, "MotionMagic"=7, "MotionProfileArc"=10, "Disabled"=15] ("Control Mode")
                    n387 = call <vilib>:"CTRE_Phoenix_MotorControl_Set.vi"("Output"=w620, "Control Mode"=w621, "PhoenixMotorControlDevRef"=w622) -> ()  [unwired: 7 in, 2 out]
                  }
                  frame True {
                  }
                }
              }
            }
          }
          frame Enabled {
            n388 = disable-structure shown="Enabled" {
              disable-tunnel: [w635 TRUE] -> w629
              disable-tunnel: [w634 TRUE] -> w628
              disable-tunnel: w625 -> [w633 _]
              frame Disabled {
                n389 = Unbundle By Name(w633) -> ("BottomRetainerSwitchDevRef"=w637:T8)
                n390 = Unbundle By Name(w633) -> ("TopRetainerSwitchDevRef"=w639:T8)
                n391 = call <vilib>:"WPI_DigitalInputGetValue.vi"("DigitalInputDevRef"=w639) -> ("Value"=w638:bool)  [unwired: 8 in, 2 out]
                n392 = call <vilib>:"WPI_DigitalInputGetValue.vi"("DigitalInputDevRef"=w637) -> ("Value"=w636:bool)  [unwired: 8 in, 2 out]
                n393 = Not(x=w636) -> (.not. x?=w634:bool)
                n394 = Not(x=w638) -> (.not. x?=w635:bool)
              }
              frame Enabled {
                # "since we aren't using the limit\nswitches now, this acts like they're\nclicked so we don't have to rewrite\neverything"
              }
            }
            n395 = Unbundle By Name(w625) -> ("Hatch Retainer States"=w632:T14)
            n396 = Unbundle By Name(w625) -> ("HatchRetainerMotorDevRef"=w630:T1)
            n397 = Unbundle By Name(w625) -> ("Hatch Retainer Move Up/Down"=w631:bool)
            n398 = case shown="\"Fully Up (retained)\"" w632 {
              tunnel: [w645 Hatch_Retainer_States."Fully Up (retained)" ("Hatch Retainer States") w655 Hatch_Retainer_States."Fully Down (not retained)" ("Hatch Retainer States")] -> w626
              tunnel: w631 -> [w648 _ w656 _]
              tunnel: w629 -> [_ _ _ _]
              tunnel: w628 -> [_ _ _ _]
              tunnel: w630 -> [w642 _ w651 _]
              tunnel: 0.2 ("Output") -> [_ _ _ _]
              frame "Fully Down (not retained)", Default {
                w644 = T33 0 items=["PercentOutput"=0, "Position"=1, "Velocity"=2, "Current"=3, "Follower"=5, "MotionProfile"=6, "MotionMagic"=7, "MotionProfileArc"=10, "Disabled"=15] ("Control Mode")
                n399 = call <vilib>:"CTRE_Phoenix_MotorControl_Set.vi"("Output"=0.0, "Control Mode"=w644, "PhoenixMotorControlDevRef"=w642) -> ()  [unwired: 7 in, 2 out]
                n400 = Select(t=Hatch_Retainer_States."Going Up" ("Hatch Retainer States"), s=w648, f=Hatch_Retainer_States."Fully Down (not retained)" ("Hatch Retainer States")) -> (s? t:f=w645:T14)
              }
              frame "Going Up" {
                # "no longer need this case since \nwe switched to a pneumatic\nretainer"
              }
              frame "Fully Up (retained)" {
                w652 = T33 0 items=["PercentOutput"=0, "Position"=1, "Velocity"=2, "Current"=3, "Follower"=5, "MotionProfile"=6, "MotionMagic"=7, "MotionProfileArc"=10, "Disabled"=15] ("Control Mode")
                n401 = call <vilib>:"CTRE_Phoenix_MotorControl_Set.vi"("Output"=0.0, "Control Mode"=w652, "PhoenixMotorControlDevRef"=w651) -> ()  [unwired: 7 in, 2 out]
                n402 = Select(t=Hatch_Retainer_States."Going Down" ("Hatch Retainer States"), s=w656, f=Hatch_Retainer_States."Fully Up (retained)" ("Hatch Retainer States")) -> (s? t:f=w655:T14)
              }
              frame "Going Down" {
                # "no longer need this case since \nwe switched to a pneumatic\nretainer"
              }
            }
          }
        }
        n403 = global read "Robot Global Data.vi" "Which Robot?"() -> (w522:T29)
        n404 = global read "Robot Global Data.vi" "Which Robot?"() -> (w521:T29)
        n405 = Unbundle By Name(w513) -> ("Hatch Collector Wanted Angle"=w516:dbl)
        n406 = Unbundle By Name(w513) -> ("Hatch Collector Actual Angle"=w515:dbl)
        n407 = case shown="\"Practice Bot\"" w521 {
          tunnel: [w732 T32 {"proportional gain (Kc)"=0.0, "integral time (Ti, min)"=0.0, "derivative time (Td, min)"=0.0} ("PID gains") T32 {"proportional gain (Kc)"=0.004, "integral time (Ti, min)"=0.0, "derivative time (Td, min)"=0.0} ("PID gains")] -> w520
          frame "Competition Bot", Default {
            # "9.7% motor speed seems\nto be minimum to move"
            n408 = disable-structure shown="Enabled" {
              disable-tunnel: [T32 {"proportional gain (Kc)"=0.03, "integral time (Ti, min)"=0.003, "derivative time (Td, min)"=0.0} ("PID gains") T32 {"proportional gain (Kc)"=0.035, "integral time (Ti, min)"=0.0, "derivative time (Td, min)"=0.0} ("PID gains")] -> w732
              frame Disabled {
              }
              frame Enabled {
              }
            }
          }
          frame "Practice Bot" {
          }
          frame "Code Bot" {
            # "p = 0.008 is WAY too fast"
            # "for code bot:\nwe ended with p = 0.004,\nbut the motor has to turn\nso slowly on the code bot\nthat no PID values would\nreally work well"
          }
        }
        n409 = case shown="\"Competition Bot\", Default" w522 {
          tunnel: [cluster{"output high":dbl, "output low":dbl} {"output high"=0.2, "output low"=-0.4} ("output range") cluster{"output high":dbl, "output low":dbl} {"output high"=0.15, "output low"=-0.15} ("output range") cluster{"output high":dbl, "output low":dbl} {"output high"=0.15, "output low"=-0.15} ("output range")] -> w514
          frame "Competition Bot", Default {
          }
          frame "Practice Bot" {
          }
          frame "Code Bot" {
          }
        }
        n410 = call-poly <vilib>:"PID.vi"("output range"=w514, "PID gains"=w520, "process variable"=w515, "setpoint"=w516) -> ("output"=w544:dbl)  [unwired: 6 in, 1 out]
        n411 = Unbundle By Name(w513) -> ("HatchCollectorMotorDevRef"=w545:T1)
        n412 = call <vilib>:"WPI_MotorControlSetOutput.vi"("Output"=w544, "MotorControlDevRef"=w545) -> ()  [unwired: 7 in, 3 out]
        n413 = Bundle By Name(cluster=w513, "Hatch Retainer States"=w524) -> (w511:T26)
      }
    }
    frame Enabled {
    }
  }
  n414 = disable-structure shown="Disabled" {
    disable-tunnel: w48 -> [w822 _]
    frame Disabled {
      # "HAB 3 Drive Module Motor"
      # "HAB 3 Pneumatics"
      # "Steps to climb HAB 3\n1. align the robot with the front of the hab 3\n2. raising up all 4 cylinders\n3. use the drive module to drive forward enough for the \n        drive train to catch the hab platform\n4. retract the front cylinders\n5. drive train and/or drive module drives forward \n         to get center of gravity over hab 3 platform\n6. raise up the back cylinders\n7. drive forward a bit more if they want\n\nWhich do we automate, and which do we have the \naux driver control manually?"
      # "Defining Global Data Values and Some Cluster Values"
      # "Defining Array Values for Joysticks"
      n415 = while {
        shift-right: [w830] -> _
        shift-left: w822 -> [w860]
        stop <- FALSE stop-if-true
        # "convert from encoder velocity to motor speed...I think"
        # "aux JS is inverted"
        n416 = Unbundle By Name(w860) -> ("DriveJoystickDevRef"=w871:T9)
        n417 = Unbundle By Name(w860) -> ("AuxJoystickDevRef"=w870:T9)
        n418 = Unbundle By Name(w860) -> ("Robot Mode"=w869:T17)
        n419 = call <vilib>:"WPI_JoystickGetValues.vi"("JoystickDevRef"=w870) -> ("Buttons"=w862:bool[], "Axes"=w863:dbl[], "JoystickDevRef"=w864:T9, "POVs"=w861:i16[])  [unwired: 6 in, 1 out]
        n420 = call <vilib>:"WPI_JoystickGetValues.vi"("JoystickDevRef"=w871) -> ("Buttons"=w866:bool[], "Axes"=w868:dbl[], "JoystickDevRef"=w867:T9, "POVs"=w865:i16[])  [unwired: 6 in, 1 out]
        n421 = Wait (ms)(milliseconds to wait=50) -> ()  [unwired: 1 out]
        n422 = case shown="\"Teleop Enabled\"" w869 {
          tunnel: w860 -> [w1050 w1060 w1061 w1062 w1072 w1073 w1074 w1084 w1085]
          tunnel: [w1050 w1051 w1061 w1063 w1072 w1073 w1074 w1075 w1085] -> w843
          tunnel: w868 -> [_ w1059 _ w1070 _ _ _ w1082 _]
          tunnel: w867 -> [_ w1058 _ w1071 _ _ _ w1083 _]
          tunnel: w866 -> [_ w1057 _ w1069 _ _ _ w1081 _]
          tunnel: w865 -> [_ w1056 _ w1068 _ _ _ w1080 _]
          tunnel: w864 -> [_ w1055 _ w1067 _ _ _ w1079 _]
          tunnel: w863 -> [_ w1054 _ w1066 _ _ _ w1078 _]
          tunnel: w862 -> [_ w1053 _ w1065 _ _ _ w1077 _]
          tunnel: w861 -> [_ w1052 _ w1064 _ _ _ w1076 _]
          frame "Autonomous Disabled", Default {
          }
          frame "Autonomous Enabled" {
            n423 = Bundle By Name(cluster=w1060, "DriveJoystickDevRef"=w1058, "Drive Axes"=w1059, "Drive Buttons"=w1057, "Drive POVs"=w1056, "AuxJoystickDevRef"=w1055, "Aux Axes"=w1054, "Aux Buttons"=w1053, "Aux POVs"=w1052) -> (w1051:T27)
          }
          frame "Teleop Disabled" {
          }
          frame "Teleop Enabled" {
            n424 = Bundle By Name(cluster=w1062, "DriveJoystickDevRef"=w1071, "Drive Axes"=w1070, "Drive Buttons"=w1069, "Drive POVs"=w1068, "AuxJoystickDevRef"=w1067, "Aux Axes"=w1066, "Aux Buttons"=w1065, "Aux POVs"=w1064) -> (w1063:T27)
          }
          frame "Disconnected" {
          }
          frame "Finish" {
          }
          frame "Test Disabled" {
          }
          frame "Test Enabled" {
            n425 = Bundle By Name(cluster=w1084, "DriveJoystickDevRef"=w1083, "Drive Axes"=w1082, "Drive Buttons"=w1081, "Drive POVs"=w1080, "AuxJoystickDevRef"=w1079, "Aux Axes"=w1078, "Aux Buttons"=w1077, "Aux POVs"=w1076) -> (w1075:T27)
          }
          frame "Emergency Stopped" {
          }
        }
        n426 = global read "Robot Global Data.vi" "Robot Mode"() -> (w845:T17)
        n427 = Bundle By Name(cluster=w843, "Robot Mode"=w845) -> (w844:T27)
        n428 = disable-structure shown="Enabled" {
          disable-tunnel: w844 -> [w976 w1020]
          disable-tunnel: w843 -> [w975 w1022]
          disable-tunnel: [_ w1007] -> w840
          frame Disabled {
            # "disabled because the RT code would override the instructions of the LT and LB code using separate bundle by names"
            # "controls both \ncylinders together"
            # "controls back cylinders only"
            # "controls front cylinders only"
            n429 = Unbundle By Name(w975) -> ("Aux Button Indexes.RT Button"=w989:i32)
            n430 = Unbundle By Name(w975) -> ("Aux Buttons"=w988:bool[])
            n431 = Unbundle By Name(w975) -> ("Aux Button Indexes.LT Button"=w991:i32)
            n432 = Unbundle By Name(w975) -> ("Front Cylinders Latch"=w984:bool)
            n433 = Unbundle By Name(w975) -> ("Aux Button Indexes.LB Button"=w1006:i32)
            n434 = Unbundle By Name(w975) -> ("Aux Buttons"=w992:bool[])
            n435 = Unbundle By Name(w975) -> ("Back Cylinders Latch"=w981:bool)
            n436 = Unbundle By Name(w975) -> ("Aux Buttons"=w1005:bool[])
            n437 = Unbundle By Name(w975) -> ("Back Cylinders Latch"=w997:bool)
            n438 = Unbundle By Name(w975) -> ("Front Cylinders Latch"=w1000:bool)
            n439 = Index Array(array=w988, index=w989) -> (element=w986:bool)
            n440 = Index Array(array=w992, index=w991) -> (element=w994:bool)
            n441 = Index Array(array=w1005, index=w1006) -> (element=w1003:bool)
            n442 = feedback #10() -> (w987:bool)  [unwired: 1 in]
            n443 = feedback-in #10(w986) -> ()
            n444 = feedback #11() -> (w993:bool)  [unwired: 1 in]
            n445 = feedback-in #11(w994) -> ()
            n446 = feedback #12() -> (w1004:bool)  [unwired: 1 in]
            n447 = feedback-in #12(w1003) -> ()
            n448 = Greater?(x=w986, y=w987) -> (0:w980:bool)
            n449 = Greater?(x=w994, y=w993) -> (0:w995:bool)
            n450 = Greater?(x=w1003, y=w1004) -> (0:w1002:bool)
            n451 = Not(x=w981) -> (.not. x?=w982:bool)
            n452 = Not(x=w984) -> (.not. x?=w985:bool)
            n453 = Not(x=w997) -> (.not. x?=w996:bool)
            n454 = Not(x=w1000) -> (.not. x?=w1001:bool)
            n455 = Select(t=w982, s=w980, f=w981) -> (s? t:f=w979:bool)
            n456 = Select(t=w985, s=w980, f=w984) -> (s? t:f=w983:bool)
            n457 = Select(t=w996, s=w995, f=w997) -> (s? t:f=w998:bool)
            n458 = Select(t=w1001, s=w1002, f=w1000) -> (s? t:f=w999:bool)
            n459 = Bundle By Name(cluster=w976, "Front Cylinders Latch"=w999) -> (w990:T27)
            n460 = Bundle By Name(cluster=w990, "Back Cylinders Latch"=w998) -> (w978:T27)
            n461 = Bundle By Name(cluster=w978, "Front Cylinders Latch"=w983) -> (w977:T27)
            n462 = Bundle By Name(cluster=w977, "Back Cylinders Latch"=w979) -> (w974:T27)
          }
          frame Enabled {
            # "controls both \ncylinders together"
            # "controls back cylinders only"
            # "controls front cylinders only"
            n463 = Unbundle By Name(w1022) -> ("Aux Button Indexes.X Button"=w1026:i32)
            n464 = Unbundle By Name(w1022) -> ("Aux Buttons"=w1025:bool[])
            n465 = Unbundle By Name(w1022) -> ("Aux Button Indexes.Y Button"=w1027:i32)
            n466 = Unbundle By Name(w1022) -> ("Aux Buttons"=w1028:bool[])
            n467 = Unbundle By Name(w1022) -> ("Aux Button Indexes.A Button"=w1034:i32)
            n468 = Unbundle By Name(w1022) -> ("Aux Buttons"=w1033:bool[])
            n469 = Unbundle By Name(w1022) -> ("Front Cylinders Latch"=w1013:bool)
            n470 = Unbundle By Name(w1022) -> ("Back Cylinders Latch"=w1010:bool)
            n471 = Index Array(array=w1025, index=w1026) -> (element=w1023:bool)
            n472 = Index Array(array=w1028, index=w1027) -> (element=w1030:bool)
            n473 = Index Array(array=w1033, index=w1034) -> (element=w1031:bool)
            n474 = feedback #13() -> (w1024:bool)  [unwired: 1 in]
            n475 = feedback-in #13(w1023) -> ()
            n476 = feedback #14() -> (w1029:bool)  [unwired: 1 in]
            n477 = feedback-in #14(w1030) -> ()
            n478 = feedback #15() -> (w1032:bool)  [unwired: 1 in]
            n479 = feedback-in #15(w1031) -> ()
            n480 = Greater?(x=w1023, y=w1024) -> (0:w1017:bool)
            n481 = Greater?(x=w1030, y=w1029) -> (0:w1018:bool)
            n482 = Greater?(x=w1031, y=w1032) -> (0:w1019:bool)
            n483 = Or(x=w1019, y=w1017) -> (x .or. y?=w1016:bool)
            n484 = Or(x=w1018, y=w1017) -> (x .or. y?=w1011:bool)
            n485 = Not(x=w1013) -> (.not. x?=w1014:bool)
            n486 = Not(x=w1010) -> (.not. x?=w1012:bool)
            n487 = Select(t=w1014, s=w1016, f=w1013) -> (s? t:f=w1015:bool)
            n488 = Select(t=w1012, s=w1011, f=w1010) -> (s? t:f=w1009:bool)
            n489 = Bundle By Name(cluster=w1020, "Front Cylinders Latch"=w1015) -> (w1021:T27)
            n490 = Bundle By Name(cluster=w1021, "Back Cylinders Latch"=w1009) -> (w1008:T27)
            n491 = disable-structure shown="Disabled" {
              disable-tunnel: w1008 -> [w1039 w1041]
              disable-tunnel: [w1038 w1041] -> w1007
              frame Disabled {
                # "yaw is the angle of our robot\npitch is the angle of elevation of our robot\nroll is how much the robot is rotated about its center"
                n492 = call <vilib>:"Get_YPRHfH.vi"() -> ("YRPHfH"=w1040:T34)  [unwired: 11 in]
                n493 = Unbundle By Name(w1040) -> ("Yaw"=w1037:dbl)
                n494 = Unbundle By Name(w1040) -> ("Pitch"=w1036:dbl)
                n495 = Unbundle By Name(w1040) -> ("Roll"=w1035:dbl)
                n496 = global write "Robot Global Data.vi" "Yaw (clockwise/counter-clockwise)"(w1037) -> ()
                n497 = global write "Robot Global Data.vi" "Roll (forward/backward tipping)"(w1035) -> ()
                n498 = global write "Robot Global Data.vi" "Pitch (left/right tipping)"(w1036) -> ()
                n499 = Bundle By Name(cluster=w1039, "Yaw"=w1037, "Pitch"=w1036, "Roll"=w1035) -> (w1038:T27)
              }
              frame Enabled {
              }
            }
          }
        }
        n500 = Unbundle By Name(w840) -> ("HAB3FrontSolenoidDevRef"=w859:T6)
        n501 = Unbundle By Name(w840) -> ("HABAssisterSolenoidDevRef"=w842:T6)
        n502 = Unbundle By Name(w840) -> ("Front Cylinders Latch"=w836:bool)
        n503 = Unbundle By Name(w840) -> ("HAB3BackSolenoidDevRef"=w853:T6)
        n504 = Unbundle By Name(w840) -> ("Back Cylinders Latch"=w835:bool)
        n505 = disable-structure shown="Disabled" {
          disable-tunnel: w835 -> [w924 _]
          disable-tunnel: w840 -> [w915 _]
          disable-tunnel: [w914 w973] -> w830
          disable-tunnel: w840 -> [w913 w973]
          frame Disabled {
            w931 = T33 2 items=["PercentOutput"=0, "Position"=1, "Velocity"=2, "Current"=3, "Follower"=5, "MotionProfile"=6, "MotionMagic"=7, "MotionProfileArc"=10, "Disabled"=15] ("Control Mode")
            # "would slow down if pos. pitch, \nwhich is opposite of what we want"
            # "base spd +- PID adjustments"
            n506 = Unbundle By Name(w915) -> ("Pitch"=w937:dbl)
            n507 = global read "Robot Global Data.vi" "Which Robot?"() -> (w935:T29)
            n508 = Unbundle By Name(w915) -> ("BkSpdAdjusterMotorDevRef"=w928:T1)
            n509 = Unbundle By Name(w915) -> ("HAB Bk Spd Motor States"=w925:T13)
            n510 = global read "Robot Global Data.vi" "Which Robot?"() -> (w933:T29)
            n511 = case shown="\"Competition Bot\", Default" w933 {
              tunnel: [cluster{"output high":dbl, "output low":dbl} {"output high"=0.2, "output low"=-0.4} ("output range") cluster{"output high":dbl, "output low":dbl} {"output high"=0.15, "output low"=-0.15} ("output range") cluster{"output high":dbl, "output low":dbl} {"output high"=0.15, "output low"=-0.15} ("output range")] -> w932
              frame "Competition Bot", Default {
              }
              frame "Practice Bot" {
              }
              frame "Code Bot" {
              }
            }
            n512 = case shown="\"Code Bot\"" w935 {
              tunnel: [T32 {"proportional gain (Kc)"=0.0, "integral time (Ti, min)"=0.0, "derivative time (Td, min)"=0.0} ("PID gains") T32 {"proportional gain (Kc)"=0.0, "integral time (Ti, min)"=0.0, "derivative time (Td, min)"=0.0} ("PID gains") T32 {"proportional gain (Kc)"=0.0, "integral time (Ti, min)"=0.0, "derivative time (Td, min)"=0.0} ("PID gains")] -> w934
              tunnel: [w967 w969 w971] -> w922
              frame "Competition Bot", Default {
                w967 = 0.0  # Enc. Val at Fully Down
              }
              frame "Practice Bot" {
                w969 = 0.0  # Enc. Val at Fully Down
              }
              frame "Code Bot" {
                w971 = 0.0  # Enc. Val at Fully Down
              }
            }
            n513 = call-poly <vilib>:"PID.vi"("output range"=w932, "PID gains"=w934, "process variable"=w937, "setpoint"=0.0) -> ("output"=w930:dbl)  [unwired: 6 in, 1 out]
            n514 = global read "Robot Global Data.vi" "HAB Bk Spd Encoder Start Value"() -> (w926:dbl)
            n515 = Negate(x=w930) -> (-x=w919:dbl)
            n516 = Add(x=w919, y=0.3) -> (x+y=w920:dbl)
            n517 = call-poly <vilib>:"CTRE_Phoenix_MotorController_Get_Enhanced.vi"("PhoenixMotorControlDevRef"=w928) -> ("Quadrature Position"=w927:i32)  [unwired: 11 in, 3 out]
            n518 = Subtract(x=w927, y=w926) -> (x-y=w916:dbl)
            n519 = Greater Or Equal?(x=w916, y=w922) -> (x >= y?=w921:bool)
            n520 = Less Or Equal To 0?(x=w916) -> (x <= 0?=w917:bool)
            n521 = case shown="\"Fully Up\", Default" w925 {
              tunnel: w924 -> [w941 _ w956 _]
              tunnel: [w942 w943 w952 w958] -> w923
              tunnel: w921 -> [_ w946 _ _]
              tunnel: w920 -> [_ w945 _ _]
              tunnel: [0.0 w944 0.0 w957] -> w918
              tunnel: w917 -> [_ _ _ w959]
              frame "Fully Up", Default {
                n522 = Select(t=HAB_Bk_Spd_Motor_States."Going Down" ("HAB Bk Spd Motor States"), s=w941, f=HAB_Bk_Spd_Motor_States."Fully Up" ("HAB Bk Spd Motor States")) -> (s? t:f=w942:T13)
              }
              frame "Going Down" {
                n523 = case shown="True" w946 {
                  tunnel: w945 -> [w948 _]
                  tunnel: [w948 0.0] -> w944
                  tunnel: [HAB_Bk_Spd_Motor_States."Going Down" ("HAB Bk Spd Motor States") HAB_Bk_Spd_Motor_States."Fully Down" ("HAB Bk Spd Motor States")] -> w943
                  frame False {
                  }
                  frame True {
                  }
                }
              }
              frame "Fully Down" {
                n524 = Not(x=w956) -> (.not. x?=w953:bool)
                n525 = Select(t=HAB_Bk_Spd_Motor_States."Going Up" ("HAB Bk Spd Motor States"), s=w953, f=HAB_Bk_Spd_Motor_States."Fully Down" ("HAB Bk Spd Motor States")) -> (s? t:f=w952:T13)
              }
              frame "Going Up" {
                n526 = case shown="True" w959 {
                  tunnel: [-0.4 0.0] -> w957
                  tunnel: [HAB_Bk_Spd_Motor_States."Going Up" ("HAB Bk Spd Motor States") HAB_Bk_Spd_Motor_States."Fully Up" ("HAB Bk Spd Motor States")] -> w958
                  frame False {
                    # "gently yeet the \nthing back up, but\nthe velocity don't\nmatter that much"
                  }
                  frame True {
                  }
                }
              }
            }
            n527 = Bundle By Name(cluster=w913, "HAB Bk Spd Motor States"=w923) -> (w914:T27)
            n528 = call <vilib>:"CTRE_Phoenix_MotorControl_Set.vi"("Output"=w918, "Control Mode"=w931, "PhoenixMotorControlDevRef"=w928) -> ()  [unwired: 7 in, 2 out]
          }
          frame Enabled {
          }
        }
        n529 = global write "Robot Global Data.vi" "HAB Back Cylinders Extended?"(w835) -> ()
        n530 = Select(t=WPI_SolenoidValue."On" ("Value"), s=w836, f=WPI_SolenoidValue."Off" ("Value")) -> (s? t:f=w841:T31)
        n531 = global write "Robot Global Data.vi" "HAB Front Cylinders Extended?"(w836) -> ()
        n532 = call-poly <vilib>:"WPI_SolenoidSet.vi"("Value"=w841, "SolenoidDevRef"=w842) -> ()  [unwired: 8 in, 2 out]
        n533 = call-poly <vilib>:"WPI_SolenoidSet.vi"("Value"=w841, "SolenoidDevRef"=w859) -> ()  [unwired: 8 in, 2 out]
        n534 = Select(t=WPI_SolenoidValue."On" ("Value"), s=w835, f=WPI_SolenoidValue."Off" ("Value")) -> (s? t:f=w856:T31)
        n535 = call-poly <vilib>:"WPI_SolenoidSet.vi"("Value"=w856, "SolenoidDevRef"=w853) -> ()  [unwired: 8 in, 2 out]
        n536 = Unbundle By Name(w830) -> ("Aux Button Indexes.B Button"=w832:i32)
        n537 = Unbundle By Name(w830) -> ("Front HAB 3 Limit Switch"=w852:T8)
        n538 = Unbundle By Name(w830) -> ("Back HAB 3 Limit Switch"=w850:T8)
        n539 = Unbundle By Name(w830) -> ("HAB3DriveModuleMotorDevRef"=w851:T1)
        n540 = Unbundle By Name(w830) -> ("Aux Buttons"=w831:bool[])
        n541 = Unbundle By Name(w830) -> ("Aux Axes"=w848:dbl[])
        n542 = Unbundle By Name(w830) -> ("Aux Joystick Indexes.Left Y"=w849:i32)
        n543 = Unbundle By Name(w830) -> ("HAB3DriveModuleMotorDevRef"=w833:T1)
        n544 = global read "Robot Global Data.vi" "Which Robot?"() -> (w837:T29)
        n545 = disable-structure shown="Disabled" {
          disable-tunnel: w830 -> [w1042 _]
          frame Disabled {
            # "maybe use in range and coerce in future to\nprevent drivers from being able to drive\nthe module backwards?"
            # "slows down motor so\nwe don't damage the\ncylinders"
            n546 = Unbundle By Name(w1042) -> ("Aux Joystick Indexes.Right Y"=w1047:i32)
            n547 = Unbundle By Name(w1042) -> ("HAB3DriveModuleMotorDevRef"=w1049:T1)
            n548 = Unbundle By Name(w1042) -> ("Aux Axes"=w1048:dbl[])
            n549 = Index Array(array=w1048, index=w1047) -> (element=w1044:dbl)
            n550 = call "Deadband.vi"("Input"=w1044) -> ("Output"=w1045:dbl)  [unwired: 10 in]
            n551 = Multiply(x=w1045, y=0.3) -> (x*y=w1043:dbl)
            n552 = call <vilib>:"WPI_MotorControlSetOutput.vi"("Output"=w1043, "MotorControlDevRef"=w1049) -> ()  [unwired: 7 in, 3 out]
          }
          frame Enabled {
          }
        }
        n553 = call <vilib>:"WPI_DigitalInputGetValue.vi"("DigitalInputDevRef"=w850) -> ("Value"=w838:bool)  [unwired: 8 in, 2 out]
        n554 = call <vilib>:"WPI_DigitalInputGetValue.vi"("DigitalInputDevRef"=w852) -> ("Value"=w839:bool)  [unwired: 8 in, 2 out]
        n555 = Index Array(array=w848, index=w849) -> (element=w846:dbl)
        n556 = Index Array(array=w831, index=w832) -> (element=w829:bool)
        n557 = case shown="\"Practice Bot\"" w837 {
          tunnel: w839 -> [w906 w910 w912]
          tunnel: [w905 w908 w912] -> w826
          tunnel: [w904 w907 w911] -> w825
          tunnel: w838 -> [w903 w909 w911]
          frame "Competition Bot", Default {
            # "they're \ninverted\nfor some \nreason?"
            n558 = Not(x=w906) -> (.not. x?=w905:bool)
            n559 = Not(x=w903) -> (.not. x?=w904:bool)
          }
          frame "Practice Bot" {
            n560 = Not(x=w910) -> (.not. x?=w908:bool)
            n561 = Not(x=w909) -> (.not. x?=w907:bool)
          }
          frame "Code Bot" {
          }
        }
        n562 = call-poly <vilib>:"CTRE_Phoenix_MotorController_Get_Enhanced.vi"("PhoenixMotorControlDevRef"=w833) -> ("Quadrature Velocity"=w824:i32)  [unwired: 11 in, 3 out]
        n563 = Negate(x=w846) -> (-x=w834:dbl)
        n564 = disable-structure shown="Enabled" {
          disable-tunnel: w824 -> [w876 w877]
          disable-tunnel: [w875 w877] -> w823
          frame Disabled {
            n565 = Divide(x=w876, y=833) -> (x/y=w875:dbl)
          }
          frame Enabled {
          }
        }
        n566 = Or(x=w826, y=w825) -> (x .or. y?=w847:bool)
        n567 = case shown="True" w829 {
          tunnel: w851 -> [w880 w894]
          tunnel: w847 -> [w879 _]
          tunnel: w834 -> [w878 w895]
          frame False {
            n568 = case shown="False" w879 {
              tunnel: w880 -> [w882 w892]
              tunnel: w878 -> [w886 _]
              frame False {
                # "negate the negated JS so it goes forward"
                # "This is a range and coerce. :P \nSees if the joystick is going backwards.\n(If the value is negative).\nIf yes, then output is set to 0.\nIf no, then output is set from the aux\njoystick. \nWe don't want the robot to go \nbackwards off of the platform. LOL"
                # "Slows down the motor output\nso we don't damage the cylinders"
                n569 = call "Deadband.vi"("Input"=w886) -> ("Output"=w890:dbl)  [unwired: 10 in]
                n570 = In Range and Coerce(upper limit=0.0, x=w886, lower limit=-1.0) -> (In Range?=w885:bool)  [unwired: 1 out]
                n571 = Multiply(x=w890, y=0.3) -> (x*y=w881:dbl)
                n572 = Select(t=0.0, s=w885, f=w881) -> (s? t:f=w884:dbl)
                n573 = call <vilib>:"WPI_MotorControlSetOutput.vi"("Output"=w884, "MotorControlDevRef"=w882) -> ()  [unwired: 7 in, 3 out]
              }
              frame True {
                # "If either the \"Front HAB 3 Limit Switch\" or \"Front HAB 3 Limit Switch\"\nis pressed, the HAB 3 Drive Module set output will be \"0.\" \n- Preventing the DRIVER from moving too far forward into\nthe HAB 3 Platform, which can damage the cylinders.\n\nIf not, the aux joysick will control the set output.\n- Enabling the DRIVER to drive forward until the robot reaches the\nplatform"
                n574 = call <vilib>:"WPI_MotorControlSetOutput.vi"("Output"=0.0, "MotorControlDevRef"=w892) -> ()  [unwired: 7 in, 3 out]
              }
            }
          }
          frame True {
            # "if da B button is pressed, then\nit overrides the switches and\nallows the HAB Drive Mod to \ngo forward. :D!!"
            # "negate the negated JS so it goes forward"
            # "This is a range and coerce. :P \nSees if the joystick is going backwards.\n(If the value is negative).\nIf yes, then output is set to 0.\nIf no, then output is set from the aux\njoystick. \nWe don't want the robot to go \nbackwards off of the platform. LOL"
            # "Slows down the motor output\nso we don't damage the cylinders"
            n575 = call "Deadband.vi"("Input"=w895) -> ("Output"=w902:dbl)  [unwired: 10 in]
            n576 = In Range and Coerce(upper limit=0.0, x=w895, lower limit=-1.0) -> (In Range?=w898:bool)  [unwired: 1 out]
            n577 = Multiply(x=w902, y=0.3) -> (x*y=w893:dbl)
            n578 = Select(t=0.0, s=w898, f=w893) -> (s? t:f=w897:dbl)
            n579 = call <vilib>:"WPI_MotorControlSetOutput.vi"("Output"=w897, "MotorControlDevRef"=w894) -> ()  [unwired: 7 in, 3 out]
          }
        }
        n580 = global write "Robot Global Data.vi" "HAB Module Actual Velocity"(w823) -> ()
        n581 = call-poly <vilib>:"NT Write Value.vi"("Boolean"=w826, "Name"="Front HAB 3 Limit Switch") -> ()  [unwired: 9 in, 1 out]
        n582 = call-poly <vilib>:"NT Write Value.vi"("Boolean"=w825, "Name"="Back HAB 3 Limit Switch") -> ()  [unwired: 9 in, 1 out]
      }
    }
    frame Enabled {
    }
  }
  n583 = disable-structure shown="Enabled" {
    frame Disabled {
      # "collector \nangle \nup/down"
      # "HAB 3 drive\nmodule"
      # "RJ"
      # "LJ"
      # "angle preset hover\nfor dust pan"
      # "angle preset out/down"
      # "angle preset in/up"
      # "lift hatch"
      # "retain hatch"
      # "kick hatch"
      # "RB"
      # "RT"
      # "LB"
      # "LT"
      # "back cylinders only"
      # "both cylinders"
      # "front cylinders only"
      # "x"
      # "a"
      # "b"
      # "y"
    }
    frame Disabled {
      # "inaccurate"
      # "collector \nangle \nup/down."
      # "HAB 3 drive\nmodule."
      # "RJ"
      # "LJ"
      # "angle preset hover\nfor dust pan."
      # "angle preset out/down"
      # "angle preset in/up."
      # "lift hatch."
      # "retain hatch."
      # "kick hatch."
      # "RB"
      # "RT"
      # "LB"
      # "LT"
      # "back cylinders only."
      # "both cylinders."
      # "front cylinders only."
      # "x"
      # "a"
      # "b"
      # "y"
    }
    frame Enabled {
    }
  }
  n584 = call "Reset Drive Encoders.vi"() -> ()  [unwired: 12 in]
  "error out" <- "error in"
